vi "Main.vi"() -> ()   [LabVIEW 2024]
uses:
  AD2_WFG_SDK_class/WFG.ctl
  AD2_WFG_SDK_class/WFGCh.ctl
  AD2_WFG_SDK_class/AD2TriggerSources.ctl
  Hamamatsu_class/SubRegion.ctl
  REGLO Digital/Controlling_the_Pump_Reglo_D.ctl
  AD2_DO_SDK_class/DOConfigureCustomData.ctl
  AD2_DO_SDK_class/DOTrigger.ctl
  AD2_DO_SDK_class/DOCustomData.ctl
  Application_class/Application.lvclass
  Users/Lab user/AppData/Local/CETONI_SDK/lib/labview/labbCAN_Bus_API/SiUnitPrefix.ctl
  Users/Lab user/AppData/Local/CETONI_SDK/lib/labview/labbCAN_Bus_API/TimeUnits.ctl
  Users/Lab user/AppData/Local/CETONI_SDK/lib/labview/labbCAN_Pump_API/VolumeUnits.ctl
  CetoniPump_class/CetoniPump.lvclass
  Cetoni_Simulated_class/Cetoni_Simulated.lvclass
  C:/git/thermacoustics/CetoniPump_class/CetoniPump.lvclass
  Hamamatsu_class/Hamamatsu.lvclass
  Hamamatsu_simulated_class/Hamamatsu_simulated.lvclass
  C:/git/thermacoustics/Hamamatsu_class/Hamamatsu.lvclass
  ExperimentSeries2_class/ExperimentSeries2.lvclass
  Valve_class/Valve.lvclass
  Valve_Sim_class/Valve_Sim.lvclass
  C:/git/thermacoustics/Valve_class/Valve.lvclass
  <vilib>/Utility/error.llb/Error Cluster From Error Code.vi
  <vilib>/ErrorRing/Error Ring.xnode
  AD2_SDK_class/AD2_SDK.lvclass
  Prior_Zmotor_class/Prior_Zmotor.lvclass
  Users/Lab user/AppData/Local/CETONI_SDK/lib/labview/labbCAN_Pump_API/labbCAN_Pump_API.lvlib
  Users/Lab user/AppData/Local/CETONI_SDK/lib/labview/labbCAN_Bus_API/labbCAN_Bus_API.lvlib
  AD2_WFG_SDK_class/AD2_WFG_SDK.lvclass
  AD2_DO_SDK_class/AD2_DO_SDK.lvclass
panel:
  in  "Abort":bool
  out "Error Out":errorcluster
  in  "Tab Control":T1(tab)=enum."Experiment"
  in  "Cetoni Device Configuration Path":string="C:\\Users\\Lab user\\Desktop\\Franzi\\Cetoni_1pump_config_FM"
  in  "Valve  VISA resource name":refnum<visa-resource-name>="COM5"
  in  "Prior Visa resource name":refnum<visa-resource-name>="COM7"
  in  "Simulate Camera":bool
  in  "Simulate Valve":bool
  in  "Simulate Pump":bool
  in  "Initialize System":bool
  in  "Z stage":bool
  in  "Analog Discovery 3":bool=TRUE
  in  "Hamamatsu":bool=TRUE
  in  "Cetoni Pump":bool=TRUE
  in  "MX Valve 2":bool=TRUE
  in  "WFGConfig":T2={"Running"=TRUE, "Ch1"={"idxChannel"=0, "Settings out of range"=FALSE, "Carrier"={"Frequency (Hz)"=1975000.0, "Amplitude (V)"=2.0, "Offset(V)"=0.0, "Symmetry(%) "=50.0, "Phase(Deg)"=0.0, "Function"=1, "Enable"=FALSE}, "Trigger"={"secRun(0=Cont)"=0.0, "secWait"=0.0, "cRepeat(0=inf)"=0, "Repeat Trigger"=FALSE, "TrigrSrc"=enum."trigrsrcNone"}, "FM Mod"={"Frequency (Hz)"=1000.0, "Amplitude (%)"=1.0, "Offset(V)"=0.0, "Symmetry(%) "=50.0, "Phase(Deg)"=0.0, "Function 2"=1, "Enable"=FALSE}}, "Ch2"={"idxChannel"=1, "Settings out of range"=FALSE, "Carrier"={"Frequency (Hz)"=1000.0, "Amplitude (V)"=1.0, "Offset(V)"=0.0, "Symmetry(%) "=50.0, "Phase(Deg)"=0.0, "Function"=1, "Enable"=FALSE}, "Trigger"={"secRun(0=Cont)"=0.0, "secWait"=0.0, "cRepeat(0=inf)"=0, "Repeat Trigger"=FALSE, "TrigrSrc"=enum."trigrsrcNone"}, "FM Mod"={"Frequency (Hz)"=1000.0, "Amplitude (%)"=1.0, "Offset(V)"=0.0, "Symmetry(%) "=50.0, "Phase(Deg)"=0.0, "Function 2"=1, "Enable"=FALSE}}, "SyncronizeState"=enum."Independent"} {"Ch2"."FM Mod"."Function 2" items=["DC"=0, "Sine"=1, "Square"=2, "Triangle"=3, "RampUp"=4, "RampDown"=5, "Noise"=6, "Pulse"=7, "Custom"=30]; "Ch2"."Carrier"."Function" items=["DC"=0, "Sine"=1, "Square"=2, "Triangle"=3, "RampUp"=4, "RampDown"=5, "Noise"=6, "Pulse"=7, "Custom"=30]; "Ch1"."FM Mod"."Function 2" items=["DC"=0, "Sine"=1, "Square"=2, "Triangle"=3, "RampUp"=4, "RampDown"=5, "Noise"=6, "Pulse"=7, "Custom"=30]; "Ch1"."Carrier"."Function" items=["DC"=0, "Sine"=1, "Square"=2, "Triangle"=3, "RampUp"=4, "RampDown"=5, "Noise"=6, "Pulse"=7, "Custom"=30]; "Ch1"."Carrier"."Frequency (Hz)" step=5000.0}
  in  "Freq Sweep (Ch1)":T5
  in  "Read Pump Status":bool
  in  "Number of flushes":dbl=2.0
  in  "Valve Pos1":bool
  in  "ValvePos2":bool
  in  "Command":T6=enum."Stop Reglo Digital"
  in  "Send Pump Command":bool
  in  "Flush":bool
  in  "Refill":bool
  in  "Flow Rate":dbl=-5000.0
  in  "Go to Level":bool
  in  "Level(ml)":dbl
  in  "Generate Flow":bool
  in  "Empty":bool
  in  "ConfigureSyringe":bool
  in  "Flush":bool
  in  "Reference move":bool
  in  "Stop Syringe":bool
  in  "Syringe":T7(ring)=enum."BD 5ml"
  in  "Flush Settings":T8={"Flush Flowrate"=1000.0, "flush volume (ml)"=0.01, "WaitAfterFlush"=5.0}
  out "Fill Level":dbl
  out "Is pumping":bool
  out "Actual Flow Rate":dbl
  in  "Adjust Intensity in image":bool
  in  "Image Continous":bool=TRUE
  in  "Center ROI":bool
  in  "ExposureTime(ms)":dbl=40.0
  in  "ROI":T9={"Horizontal Offset"=0, "Vertical Offset"=792, "Horizontal Size"=2304, "Vertical Size"=740} {"Vertical Size" min=4 max=1512 step=4; "Horizontal Size" min=4 max=2304 step=4; "Vertical Offset" min=0 max=1564 step=4; "Horizontal Offset" min=0 max=0 step=4}
  in  "Image":bool
  in  "Configure Camera":bool
  in  "Trigg":bool
  out "Frame Index 2":i32
  out "Frame Count 2":i32
  in  "StartSequence":bool
  in  "SaveSequence":bool
  in  "Sequence path":path
  in  "Sequence Settings":T10={"Master Pulse Settings"={"Mode"=1, "Source"=1, "Interval"=1.0, "Burst"=0}, "Capture mode"=0, "Frames"=0, "Dcam Trigger Source"=1, "External Options"={"Polarity"=1, "Delay"=0.0}, "ExposureTime(ms)"=0.0} {"External Options"."Polarity" items=["Negative"=1, "Positive"=2]; "Dcam Trigger Source" items=["Internal"=1, "External"=2, "Software"=3, "Master Pulse"=4]; "Capture mode" items=["Snap", "Sequence"]; "Master Pulse Settings"."Source" items=["External"=1, "Software"=2]; "Master Pulse Settings"."Mode" items=["Continuous"=1, "Start"=2, "Burst"=3]}
  in  "Conversion Policy (Default)":T11={"Conversion Method"=15, "Minimum Value"=0, "Maximum Value"=0, "# Shifts"=0} {"Conversion Method" items=["Default"=10, "Most Significant Bits"=11, "Full Dynamic"=12, "Downshift"=13, "Given Range"=14, "90% Dynamic"=15, "Given Percent Range"=16]}
  in  "?":T12={"DO Trigger"={"secRun(0=Cont)"=0.0, "secWait"=0.0, "cRepeat(0=inf)"=0, "Repeat Trigger"=FALSE, "TrigrSrc"=enum."trigrsrcNone"}, "CustomData"=[{"Data"=[FALSE, TRUE, FALSE, FALSE, FALSE, FALSE, FALSE, FALSE, FALSE, FALSE, FALSE, FALSE, FALSE, FALSE, FALSE, FALSE, FALSE, FALSE, FALSE, FALSE, FALSE, FALSE], "Freq"=1000.0, "#Bits"=100, "Enable"=FALSE, "IdleState"=0}, {"Data"=[TRUE, TRUE, TRUE, TRUE, TRUE, FALSE, FALSE, FALSE, FALSE, FALSE, FALSE, FALSE, FALSE, FALSE, FALSE, FALSE, FALSE, FALSE, FALSE, FALSE, FALSE, FALSE], "Freq"=1000.0, "#Bits"=100, "Enable"=FALSE, "IdleState"=0}, {"Data"=[], "Freq"=0.0, "#Bits"=0, "Enable"=FALSE, "IdleState"=0}, {"Data"=[FALSE, FALSE, FALSE, FALSE, FALSE, FALSE, FALSE, FALSE, FALSE, FALSE, FALSE, FALSE, FALSE, FALSE, FALSE, FALSE, FALSE, FALSE, FALSE, FALSE, FALSE, FALSE, FALSE], "Freq"=0.0, "#Bits"=0, "Enable"=FALSE, "IdleState"=0}, {"Data"=[], "Freq"=0.0, "#Bits"=0, "Enable"=FALSE, "IdleState"=0}, {"Data"=[], "Freq"=0.0, "#Bits"=0, "Enable"=FALSE, "IdleState"=0}, {"Data"=[], "Freq"=0.0, "#Bits"=0, "Enable"=FALSE, "IdleState"=0}, {"Data"=[], "Freq"=0.0, "#Bits"=0, "Enable"=FALSE, "IdleState"=0}, {"Data"=[], "Freq"=0.0, "#Bits"=0, "Enable"=FALSE, "IdleState"=0}, {"Data"=[], "Freq"=0.0, "#Bits"=0, "Enable"=FALSE, "IdleState"=0}, {"Data"=[], "Freq"=0.0, "#Bits"=0, "Enable"=FALSE, "IdleState"=0}, {"Data"=[], "Freq"=0.0, "#Bits"=0, "Enable"=FALSE, "IdleState"=0}, {"Data"=[], "Freq"=0.0, "#Bits"=0, "Enable"=FALSE, "IdleState"=0}, {"Data"=[], "Freq"=0.0, "#Bits"=0, "Enable"=FALSE, "IdleState"=0}, {"Data"=[], "Freq"=0.0, "#Bits"=0, "Enable"=FALSE, "IdleState"=0}, {"Data"=[FALSE, FALSE, FALSE, FALSE, FALSE, FALSE, FALSE, FALSE, FALSE, FALSE, FALSE, FALSE, FALSE, FALSE, FALSE, FALSE, FALSE, FALSE, FALSE, FALSE, FALSE, FALSE, FALSE], "Freq"=0.0, "#Bits"=0, "Enable"=FALSE, "IdleState"=0}, {"Data"=[FALSE, FALSE, FALSE, FALSE, FALSE, FALSE, FALSE, FALSE, FALSE, FALSE, FALSE, FALSE, FALSE, FALSE, FALSE, FALSE, FALSE, FALSE, FALSE, FALSE, FALSE, FALSE, FALSE], "Freq"=0.0, "#Bits"=0, "Enable"=FALSE, "IdleState"=0}]}
  in  "Configure DO":bool
  in  "Configure DO Clock":bool
  in  "DO Trigger":T13
  in  "ClockSettings":T15(array[cluster])
  in  "TriggAD2":bool
  in  "Frequency List Generator":bool
  in  "Frequency List":dbl[](array[numeric])=[0.0, 1.0]
  in  "Dynamic Frequency \n(or center freq)":bool
  in  "SeriesPath 2":path=path "D:/2026-02-17_Rev_Strea_OffcLaser_1micr/1975kHz/1500mMol_20C_test2"
  in  "Start Experiment series":bool
  out "# elements in queue":i32=1
  out "Time Left":dbl=inf format="%<%H:%M:%S>t"
  out "Elapsed Time":dbl=6.602530002593994 format="%<%H:%M:%S>t"
  in  "Frames":i32=1000 min=1
  in  "ExposureTime(ms) 2":dbl=40.0
  in  "Repeats":i32=1 min=1
  in  "Flush Settings 2":T16={"Flush Flowrate(uL)"=1000.0, "flush volume (ml)"=0.01, "WaitAfterFlush"=2.0}
  out "Waveform Graph":dbl[](graph)=[0.04999995231628418, 0.05000019073486328, 0.050000905990600586, 0.04999995231628418, 0.05000114440917969, 0.04999995231628418, 0.050000905990600586, 0.04999995231628418, 0.05000114440917969, 0.04999995231628418, 0.050000905990600586, 0.05000019073486328, 0.050000905990600586, 0.04999995231628418, 0.05000114440917969, 0.04999995231628418, 0.050000905990600586, 0.04999995231628418, 0.049996137619018555, 0.04999995231628418, 0.050000905990600586, 0.05000019073486328, 0.04999995231628418, 0.050000905990600586, 0.04999995231628418, 0.05000114440917969, 0.04999995231628418, 0.050000905990600586, 0.05000019073486328, 0.050000905990600586, 0.04999995231628418, 0.05000114440917969, 0.04999995231628418, 0.050000905990600586, 0.04999995231628418, 0.05000114440917969, 0.04999995231628418, 0.050000905990600586, 0.05000019073486328, 0.04999589920043945, 0.04999995231628418, 0.05000114440917969, 0.04999995231628418, 0.04999995231628418, 0.050000905990600586, 0.05000019073486328, 0.050000905990600586, 0.04999995231628418, 0.05000114440917969, 0.04999995231628418, 0.050000905990600586, 0.04999995231628418, 0.05000114440917969, 0.04999995231628418, 0.050000905990600586, 0.05000019073486328, 0.050000905990600586, 0.04999995231628418, 0.05000114440917969, 0.04999995231628418, 0.04999589920043945, 0.04999995231628418, 0.05000114440917969, 0.04999995231628418, 0.04999995231628418, 0.05000114440917969, 0.04999995231628418, 0.050000905990600586, 0.04999995231628418, 0.05000114440917969, 0.04999995231628418, 0.050000905990600586, 0.05000019073486328, 0.050000905990600586, 0.04999995231628418, 0.050000905990600586, 0.05000019073486328, 0.050000905990600586, 0.04999995231628418, 0.05000114440917969, 0.04999995231628418, 0.04999589920043945, 0.05000019073486328, 0.050000905990600586, 0.04999995231628418, 0.050000905990600586, 0.05000019073486328, 0.04999995231628418, 0.050000905990600586, 0.04999995231628418, 0.05000114440917969, 0.04999995231628418, 0.050000905990600586, 0.05000019073486328, 0.050000905990600586, 0.04999995231628418, 0.05000114440917969, 0.04999995231628418, 0.050000905990600586, 0.04999995231628418, 0.05000114440917969, 0.04999995231628418, 0.04999589920043945, 0.05000019073486328, 0.050000905990600586, 0.04999995231628418, 0.05000114440917969, 0.04999995231628418, 0.04999995231628418, 0.050000905990600586, 0.05000019073486328, 0.050000905990600586, 0.04999995231628418, 0.05000114440917969, 0.04999995231628418, 0.050000905990600586, 0.04999995231628418, 0.05000114440917969, 0.04999995231628418, 0.050000905990600586, 0.05000019073486328, 0.050000905990600586, 0.04999995231628418, 0.049996137619018555, 0.04999995231628418, 0.050000905990600586, 0.04999995231628418, 0.05000114440917969, 0.04999995231628418, 0.04999995231628418, 0.05000114440917969, 0.04999995231628418, 0.050000905990600586, 0.04999995231628418, 0.05000114440917969, 0.04999995231628418, 0.050000905990600586, 0.05000019073486328, 0.050000905990600586, 0.04999995231628418, 0.05000114440917969, 0.04999995231628418, 0.050000905990600586, 0.04999494552612305, 0.05000114440917969, 0.04999995231628418, 0.050000905990600586, 0.05000019073486328, 0.050000905990600586, 0.04999995231628418, 0.04999995231628418, 0.05000114440917969, 0.04999995231628418, 0.050000905990600586, 0.05000019073486328, 0.050000905990600586, 0.04999995231628418, 0.05000114440917969, 0.04999995231628418, 0.050000905990600586, 0.04999995231628418, 0.05000114440917969, 0.04999995231628418, 0.050000905990600586, 0.04999518394470215, 0.050000905990600586, 0.04999995231628418, 0.05000114440917969, 0.04999995231628418, 0.050000905990600586, 0.04999995231628418, 0.05000114440917969, 0.04999995231628418, 0.04999995231628418, 0.05000114440917969, 0.04999995231628418, 0.050000905990600586, 0.04999995231628418, 0.05000114440917969, 0.04999995231628418, 0.050000905990600586, 0.05000019073486328, 0.050000905990600586, 0.04999995231628418, 0.05000114440917969, 0.04999494552612305, 0.050000905990600586, 0.04999995231628418, 0.05000114440917969, 0.04999995231628418, 0.050000905990600586, 0.05000019073486328, 0.050000905990600586, 0.04999995231628418, 0.04999995231628418, 0.05000114440917969, 0.04999995231628418, 0.050000905990600586, 0.05000019073486328, 0.050000905990600586, 0.04999995231628418, 0.05000114440917969, 0.04999995231628418, 0.050000905990600586, 0.04999995231628418, 0.049996137619018555, 0.04999995231628418, 0.050000905990600586, 0.05000019073486328, 0.050000905990600586, 0.04999995231628418, 0.05000114440917969, 0.04999995231628418, 0.050000905990600586, 0.04999995231628418, 0.05000019073486328, 0.050000905990600586, 0.04999995231628418, 0.05000114440917969, 0.04999995231628418, 0.050000905990600586, 0.04999995231628418, 0.05000114440917969, 0.04999995231628418, 0.050000905990600586, 0.04999518394470215, 0.050000905990600586, 0.04999995231628418, 0.05000114440917969, 0.04999995231628418, 0.050000905990600586, 0.04999995231628418, 0.05000114440917969, 0.04999995231628418, 0.050000905990600586, 0.04999995231628418, 0.05000019073486328, 0.050000905990600586, 0.04999995231628418, 0.05000114440917969, 0.04999995231628418, 0.050000905990600586, 0.04999995231628418, 0.05000114440917969, 0.04999995231628418, 0.04999589920043945, 0.05000019073486328, 0.050000905990600586, 0.04999995231628418, 0.05000114440917969, 0.04999995231628418, 0.050000905990600586, 0.04999995231628418, 0.05000114440917969, 0.04999995231628418, 0.050000905990600586, 0.05000019073486328, 0.050000905990600586, 0.04999995231628418, 0.04999995231628418, 0.05000114440917969, 0.04999995231628418, 0.050000905990600586, 0.05000019073486328, 0.050000905990600586, 0.04999995231628418, 0.049996137619018555, 0.04999995231628418, 0.050000905990600586, 0.04999995231628418, 0.05000114440917969, 0.04999995231628418, 0.050000905990600586, 0.05000019073486328, 0.050000905990600586, 0.04999995231628418, 0.05000114440917969, 0.04999995231628418, 0.050000905990600586, 0.04999995231628418, 0.05000019073486328, 0.050000905990600586, 0.04999995231628418, 0.05000114440917969, 0.04999995231628418, 0.050000905990600586, 0.04999995231628418, 0.049996137619018555, 0.04999995231628418, 0.050000905990600586, 0.05000019073486328, 0.050000905990600586, 0.04999995231628418, 0.05000114440917969, 0.04999995231628418, 0.050000905990600586, 0.04999995231628418, 0.05000114440917969, 0.04999995231628418, 0.050000905990600586, 0.05000019073486328, 0.04999995231628418, 0.050000905990600586, 0.04999995231628418, 0.05000114440917969, 0.04999995231628418, 0.050000905990600586, 0.05000019073486328, 0.04999589920043945, 0.04999995231628418, 0.05000114440917969, 0.04999995231628418, 0.050000905990600586, 0.04999995231628418, 0.05000114440917969, 0.04999995231628418, 0.050000905990600586, 0.05000019073486328, 0.050000905990600586, 0.04999995231628418, 0.05000114440917969, 0.04999995231628418, 0.04999995231628418, 0.050000905990600586, 0.05000019073486328, 0.050000905990600586, 0.04999995231628418, 0.05000114440917969, 0.04999494552612305, 0.050000905990600586, 0.04999995231628418, 0.05000114440917969, 0.04999995231628418, 0.050000905990600586, 0.05000019073486328, 0.050000905990600586, 0.04999995231628418, 0.05000114440917969, 0.04999995231628418, 0.050000905990600586, 0.04999995231628418, 0.05000114440917969, 0.04999995231628418, 0.050000905990600586, 0.05000019073486328, 0.04999995231628418, 0.050000905990600586, 0.04999995231628418, 0.05000114440917969, 0.04999494552612305, 0.050000905990600586, 0.05000019073486328, 0.050000905990600586, 0.04999995231628418, 0.05000114440917969, 0.04999995231628418, 0.050000905990600586, 0.04999995231628418, 0.05000114440917969, 0.04999995231628418, 0.050000905990600586, 0.05000019073486328, 0.050000905990600586, 0.04999995231628418, 0.05000114440917969, 0.04999995231628418, 0.04999995231628418, 0.050000905990600586, 0.04999995231628418, 0.049996137619018555, 0.04999995231628418, 0.05000114440917969, 0.04999995231628418, 0.050000905990600586, 0.04999995231628418, 0.05000114440917969, 0.04999995231628418, 0.050000905990600586, 0.04999995231628418, 0.05000114440917969, 0.04999995231628418, 0.050000905990600586, 0.05000019073486328, 0.050000905990600586, 0.04999995231628418, 0.05000114440917969, 0.04999995231628418, 0.04999995231628418, 0.050000905990600586, 0.05000019073486328, 0.04999589920043945, 0.04999995231628418, 0.05000114440917969, 0.04999995231628418, 0.050000905990600586, 0.04999995231628418, 0.05000114440917969, 0.04999995231628418, 0.050000905990600586, 0.05000019073486328, 0.050000905990600586, 0.04999995231628418, 0.05000114440917969, 0.04999995231628418, 0.050000905990600586, 0.04999995231628418, 0.05000114440917969, 0.04999995231628418, 0.04999995231628418, 0.05000114440917969, 0.04999995231628418, 0.050000905990600586, 0.049996137619018555, 0.04999995231628418, 0.04999995231628418, 0.050000905990600586, 0.05000019073486328, 0.050000905990600586, 0.04999995231628418, 0.05000114440917969, 0.04999995231628418, 0.050000905990600586, 0.04999995231628418, 0.05000114440917969, 0.04999995231628418, 0.050000905990600586, 0.05000019073486328, 0.050000905990600586, 0.04999995231628418, 0.05000114440917969, 0.04999995231628418, 0.04999995231628418, 0.050000905990600586, 0.049996137619018555, 0.04999995231628418, 0.04999995231628418, 0.05000114440917969, 0.04999995231628418, 0.050000905990600586, 0.04999995231628418, 0.05000114440917969, 0.04999995231628418, 0.050000905990600586, 0.05000019073486328, 0.050000905990600586, 0.04999995231628418, 0.05000114440917969, 0.04999995231628418, 0.050000905990600586, 0.04999995231628418, 0.05000114440917969, 0.04999995231628418, 0.04999995231628418, 0.05000114440917969, 0.04999589920043945, 0.04999995231628418, 0.04999995231628418, 0.05000114440917969, 0.04999995231628418, 0.050000905990600586, 0.05000019073486328, 0.050000905990600586, 0.04999995231628418, 0.05000114440917969, 0.04999995231628418, 0.050000905990600586, 0.04999995231628418, 0.05000114440917969, 0.04999995231628418, 0.050000905990600586, 0.05000019073486328, 0.050000905990600586, 0.04999995231628418, 0.04999995231628418, 0.049996137619018555, 0.050000905990600586, 0.04999995231628418, 0.05000019073486328, 0.050000905990600586, 0.04999995231628418, 0.05000114440917969, 0.04999995231628418, 0.050000905990600586, 0.04999995231628418, 0.05000114440917969, 0.04999995231628418, 0.050000905990600586, 0.05000019073486328, 0.050000905990600586, 0.04999995231628418, 0.05000114440917969, 0.04999995231628418, 0.050000905990600586, 0.04999995231628418, 0.05000019073486328, 0.04999589920043945, 0.050000905990600586, 0.05000019073486328, 0.050000905990600586, 0.04999995231628418, 0.04999995231628418, 0.05000114440917969, 0.04999995231628418, 0.050000905990600586, 0.05000019073486328, 0.050000905990600586, 0.04999995231628418, 0.05000114440917969, 0.04999995231628418, 0.050000905990600586, 0.04999995231628418, 0.05000114440917969, 0.04999995231628418, 0.050000905990600586, 0.04999995231628418, 0.05000114440917969, 0.04999494552612305, 0.05000114440917969, 0.04999995231628418, 0.050000905990600586, 0.04999995231628418, 0.05000019073486328, 0.050000905990600586, 0.04999995231628418, 0.050000905990600586, 0.05000019073486328, 0.050000905990600586, 0.04999995231628418, 0.05000114440917969, 0.04999995231628418, 0.050000905990600586, 0.04999995231628418, 0.05000114440917969, 0.04999995231628418, 0.050000905990600586, 0.05000019073486328, 0.050000905990600586, 0.04999494552612305, 0.05000114440917969, 0.04999995231628418, 0.050000905990600586, 0.04999995231628418, 0.05000019073486328, 0.050000905990600586, 0.04999995231628418, 0.05000114440917969, 0.04999995231628418, 0.050000905990600586, 0.04999995231628418, 0.05000114440917969, 0.04999995231628418, 0.050000905990600586, 0.05000019073486328, 0.050000905990600586, 0.04999995231628418, 0.05000114440917969, 0.04999995231628418, 0.050000905990600586, 0.04999995231628418, 0.049996137619018555, 0.04999995231628418, 0.050000905990600586, 0.05000019073486328, 0.04999995231628418, 0.050000905990600586, 0.04999995231628418, 0.05000114440917969, 0.04999995231628418, 0.050000905990600586, 0.05000019073486328, 0.050000905990600586, 0.04999995231628418, 0.05000114440917969, 0.04999995231628418, 0.050000905990600586, 0.04999995231628418, 0.05000114440917969, 0.04999995231628418, 0.050000905990600586, 0.05000019073486328, 0.04999589920043945, 0.04999995231628418, 0.05000114440917969, 0.04999995231628418, 0.050000905990600586, 0.04999995231628418, 0.05000019073486328, 0.050000905990600586, 0.04999995231628418, 0.05000114440917969, 0.04999995231628418, 0.050000905990600586, 0.04999995231628418, 0.05000114440917969, 0.04999995231628418, 0.050000905990600586, 0.05000019073486328, 0.050000905990600586, 0.04999995231628418, 0.05000114440917969, 0.04999995231628418, 0.050000905990600586, 0.04999494552612305, 0.05000114440917969, 0.04999995231628418, 0.050000905990600586, 0.05000019073486328, 0.04999995231628418, 0.050000905990600586, 0.04999995231628418, 0.05000114440917969, 0.04999995231628418, 0.050000905990600586, 0.05000019073486328, 0.050000905990600586, 0.04999995231628418, 0.05000114440917969, 0.04999995231628418, 0.050000905990600586, 0.04999995231628418, 0.05000114440917969, 0.04999995231628418, 0.050000905990600586, 0.05000019073486328, 0.04999589920043945, 0.04999995231628418, 0.05000114440917969, 0.04999995231628418, 0.04999995231628418, 0.050000905990600586, 0.05000019073486328, 0.050000905990600586, 0.04999995231628418, 0.05000114440917969, 0.04999995231628418, 0.050000905990600586, 0.04999995231628418, 0.05000114440917969, 0.04999995231628418, 0.050000905990600586, 0.05000019073486328, 0.050000905990600586, 0.04999995231628418, 0.05000114440917969, 0.04999995231628418, 0.04999589920043945, 0.04999995231628418, 0.05000114440917969, 0.04999995231628418, 0.04999995231628418, 0.05000114440917969, 0.04999995231628418, 0.050000905990600586, 0.04999995231628418, 0.05000114440917969, 0.04999995231628418, 0.050000905990600586, 0.05000019073486328, 0.050000905990600586, 0.04999995231628418, 0.050000905990600586, 0.05000019073486328, 0.050000905990600586, 0.04999995231628418, 0.05000114440917969, 0.04999995231628418, 0.04999589920043945, 0.05000019073486328, 0.050000905990600586, 0.04999995231628418, 0.050000905990600586, 0.05000019073486328, 0.04999995231628418, 0.050000905990600586, 0.04999995231628418, 0.05000114440917969, 0.04999995231628418, 0.050000905990600586, 0.05000019073486328, 0.050000905990600586, 0.04999995231628418, 0.05000114440917969, 0.04999995231628418, 0.050000905990600586, 0.04999995231628418, 0.05000114440917969, 0.04999995231628418, 0.04999589920043945, 0.05000019073486328, 0.050000905990600586, 0.04999995231628418, 0.05000114440917969, 0.04999995231628418, 0.04999995231628418, 0.050000905990600586, 0.05000019073486328, 0.050000905990600586, 0.04999995231628418, 0.05000114440917969, 0.04999995231628418, 0.050000905990600586, 0.04999995231628418, 0.05000114440917969, 0.04999995231628418, 0.050000905990600586, 0.05000019073486328, 0.050000905990600586, 0.04999995231628418, 0.049996137619018555, 0.04999995231628418, 0.050000905990600586, 0.04999995231628418, 0.05000114440917969, 0.04999995231628418, 0.04999995231628418, 0.05000114440917969, 0.04999995231628418, 0.050000905990600586, 0.04999995231628418, 0.05000114440917969, 0.04999995231628418, 0.050000905990600586, 0.05000019073486328, 0.050000905990600586, 0.04999995231628418, 0.05000114440917969, 0.04999995231628418, 0.050000905990600586, 0.04999995231628418, 0.049996137619018555, 0.04999995231628418, 0.050000905990600586, 0.05000019073486328, 0.050000905990600586, 0.04999995231628418, 0.04999995231628418, 0.05000114440917969, 0.04999995231628418, 0.050000905990600586, 0.05000019073486328, 0.050000905990600586, 0.04999995231628418, 0.05000114440917969, 0.04999995231628418, 0.050000905990600586, 0.04999995231628418, 0.05000114440917969, 0.04999995231628418, 0.050000905990600586, 0.04999518394470215, 0.050000905990600586, 0.04999995231628418, 0.05000114440917969, 0.04999995231628418, 0.050000905990600586, 0.04999995231628418, 0.05000114440917969, 0.04999995231628418, 0.04999995231628418, 0.05000114440917969, 0.04999995231628418, 0.050000905990600586, 0.04999995231628418, 0.05000114440917969, 0.04999995231628418, 0.050000905990600586, 0.05000019073486328, 0.050000905990600586, 0.04999995231628418, 0.05000114440917969, 0.04999494552612305, 0.050000905990600586, 0.04999995231628418, 0.05000114440917969, 0.04999995231628418, 0.050000905990600586, 0.05000019073486328, 0.050000905990600586, 0.04999995231628418, 0.04999995231628418, 0.05000114440917969, 0.04999995231628418, 0.050000905990600586, 0.05000019073486328, 0.050000905990600586, 0.04999995231628418, 0.05000114440917969, 0.04999995231628418, 0.050000905990600586, 0.04999995231628418, 0.049996137619018555, 0.04999995231628418, 0.050000905990600586, 0.05000019073486328, 0.050000905990600586, 0.04999995231628418, 0.05000114440917969, 0.04999995231628418, 0.050000905990600586, 0.04999995231628418, 0.05000019073486328, 0.050000905990600586, 0.04999995231628418, 0.05000114440917969, 0.04999995231628418, 0.050000905990600586, 0.04999995231628418, 0.05000114440917969, 0.04999995231628418, 0.050000905990600586, 0.04999995231628418, 0.049996137619018555, 0.04999995231628418, 0.05000114440917969, 0.04999995231628418, 0.050000905990600586, 0.04999995231628418, 0.05000114440917969, 0.04999995231628418, 0.050000905990600586, 0.04999995231628418, 0.05000019073486328, 0.050000905990600586, 0.04999995231628418, 0.05000114440917969, 0.04999995231628418, 0.050000905990600586, 0.04999995231628418, 0.05000114440917969, 0.04999995231628418, 0.050000905990600586, 0.05000019073486328, 0.04999589920043945, 0.04999995231628418, 0.05000114440917969, 0.04999995231628418, 0.050000905990600586, 0.04999995231628418, 0.05000114440917969, 0.04999995231628418, 0.050000905990600586, 0.05000019073486328, 0.050000905990600586, 0.04999995231628418, 0.04999995231628418, 0.05000114440917969, 0.04999995231628418, 0.050000905990600586, 0.05000019073486328, 0.050000905990600586, 0.04999995231628418, 0.05000114440917969, 0.04999995231628418, 0.04999589920043945, 0.04999995231628418, 0.05000114440917969, 0.04999995231628418, 0.050000905990600586, 0.05000019073486328, 0.050000905990600586, 0.04999995231628418, 0.05000114440917969, 0.04999995231628418, 0.050000905990600586, 0.04999995231628418, 0.05000019073486328, 0.050000905990600586, 0.04999995231628418, 0.05000114440917969, 0.04999995231628418, 0.050000905990600586, 0.04999995231628418, 0.049996137619018555, 0.04999995231628418, 0.050000905990600586, 0.05000019073486328, 0.050000905990600586, 0.04999995231628418, 0.05000114440917969, 0.04999995231628418, 0.050000905990600586, 0.04999995231628418, 0.05000114440917969, 0.04999995231628418, 0.050000905990600586, 0.05000019073486328, 0.04999995231628418, 0.050000905990600586, 0.04999995231628418, 0.05000114440917969, 0.04999995231628418, 0.050000905990600586, 0.04999518394470215, 0.050000905990600586, 0.04999995231628418, 0.05000114440917969, 0.04999995231628418, 0.050000905990600586, 0.04999995231628418, 0.05000114440917969, 0.04999995231628418, 0.050000905990600586, 0.05000019073486328, 0.050000905990600586, 0.04999995231628418, 0.05000114440917969, 0.04999995231628418, 0.04999995231628418, 0.050000905990600586, 0.05000019073486328, 0.050000905990600586, 0.04999995231628418, 0.049996137619018555, 0.04999995231628418, 0.050000905990600586, 0.04999995231628418, 0.05000114440917969, 0.04999995231628418, 0.050000905990600586, 0.05000019073486328, 0.050000905990600586, 0.04999995231628418, 0.05000114440917969, 0.04999995231628418, 0.050000905990600586, 0.04999995231628418, 0.05000114440917969, 0.04999995231628418, 0.050000905990600586, 0.05000019073486328, 0.04999995231628418, 0.04999589920043945, 0.05000114440917969, 0.04999995231628418, 0.04999995231628418, 0.050000905990600586, 0.05000019073486328, 0.050000905990600586, 0.04999995231628418, 0.05000114440917969, 0.04999995231628418, 0.050000905990600586, 0.04999995231628418, 0.05000114440917969, 0.04999995231628418, 0.050000905990600586, 0.05000019073486328, 0.050000905990600586, 0.04999995231628418, 0.05000114440917969, 0.04999995231628418, 0.04999995231628418, 0.04999589920043945, 0.05000114440917969, 0.04999995231628418, 0.04999995231628418, 0.05000114440917969, 0.04999995231628418, 0.050000905990600586, 0.04999995231628418, 0.05000114440917969, 0.04999995231628418, 0.050000905990600586, 0.05000019073486328, 0.050000905990600586, 0.04999995231628418, 0.050000905990600586, 0.05000019073486328, 0.050000905990600586, 0.04999995231628418, 0.05000114440917969, 0.04999995231628418, 0.04999589920043945, 0.05000019073486328, 0.050000905990600586, 0.04999995231628418, 0.04999995231628418, 0.05000114440917969, 0.04999995231628418, 0.050000905990600586, 0.04999995231628418, 0.05000114440917969, 0.04999995231628418, 0.050000905990600586, 0.05000019073486328, 0.050000905990600586, 0.04999995231628418, 0.05000114440917969, 0.04999995231628418, 0.050000905990600586, 0.04999995231628418, 0.05000114440917969, 0.04999995231628418, 0.04999995231628418, 0.049996137619018555, 0.050000905990600586, 0.04999995231628418, 0.05000114440917969, 0.04999995231628418]
  out "Average FPS":dbl=20.019925398487086
  in  "Analog Discovery Settings":T17={"Camera FPS"=20.0, "Camera Start (s)"=0.0, "Ch1 Frequency (Hz)"=1975000.0, "Ch1.Carrier.Amplitude (V)"=2.0, "Ch1 Start (s)"=0.0, "Ch1 Run (s) (0=Cont)"=60.0, "Ch2 Start(s)"=0.0, "Ch2 Run (s)(0=Cont)"=60.0}
  in  "GlobalExposure":bool
  in  "Dynamic Camera Start Time":bool
  in  "Camera Start Array(s)":dbl[](array[numeric])=[0.0, 1.0]
  in  "Freq Sweep (Ch1) 2":T5
  in  "Get Z Stack":bool
  in  "GoToPosPrior":bool
  in  "Pos (um)":i32
  in  "Read Position":bool
  in  "Top":dbl
  in  "Bottom":dbl
  in  "Step Size":dbl
  in  "Zero Z":bool
  out "Position (um)":dbl
  out "Status":string="FlushComplete"
  in  "Exit":bool
  # "If Freq Sweep Is enabled, it overrides ch1 frequency"
  # "Sweep Span=Freq Stop-Freq Start\nFreq start=Center Freq- 1/2 Freq Span\nCenter Freq = Ch1 Freq or Frequency List"
  # "These Go MAX flow!"
  # "476 is Vertical is max for 100 fps"
  # "0 init\n1 low\n2 high\n3 tristate"
  # "Sweep Span=Freq Stop-Freq Start\nFreq start=Center Freq- 1/2 Freq Span\nCenter Freq = Ch1 Freq or Frequency List"
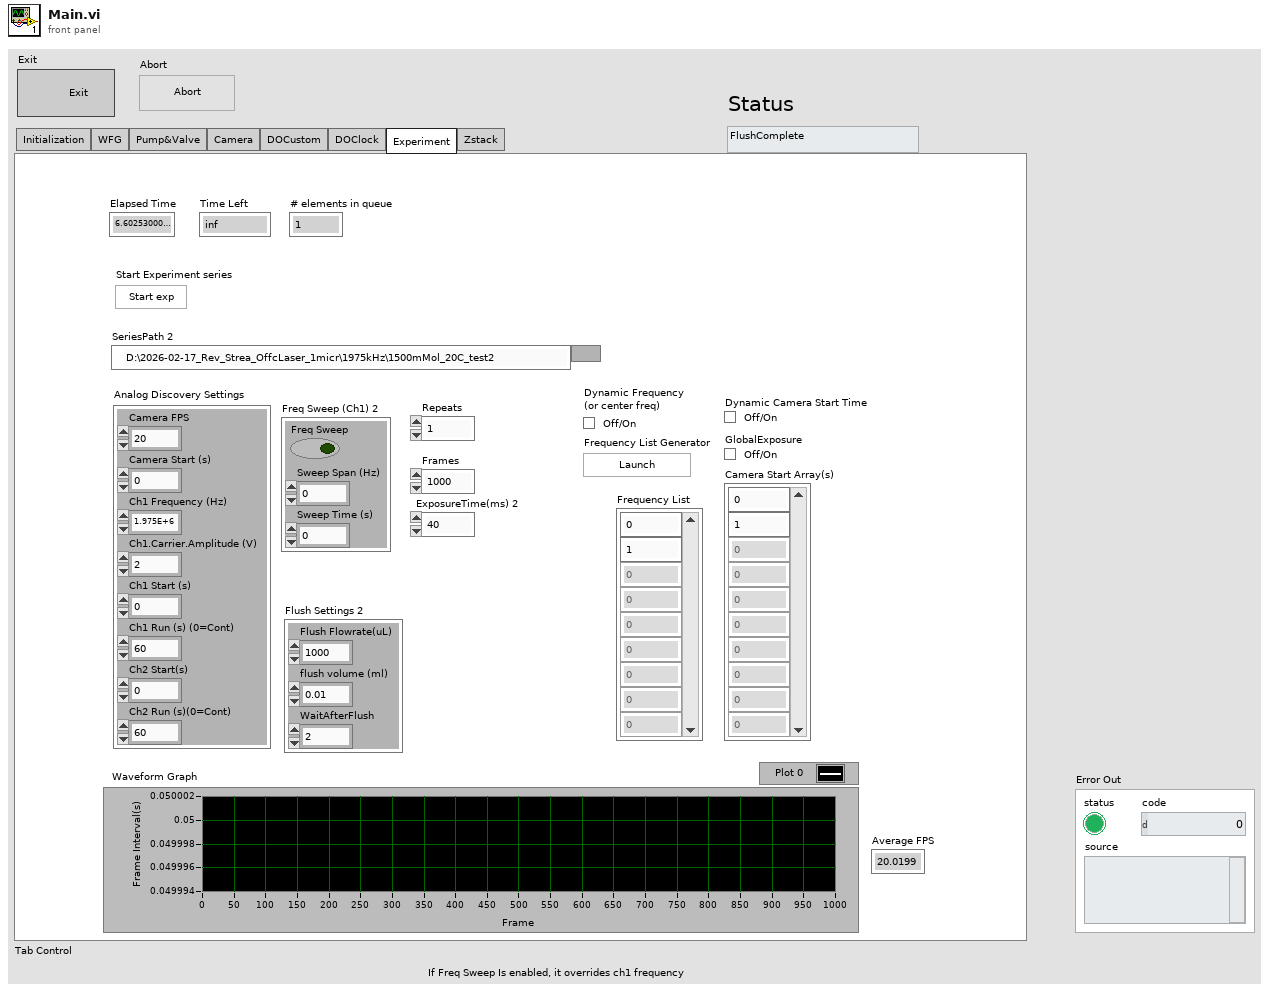
[diagram p1: front panel]
types:
  T1 = enum32{"Initialization", "WFG", "Pump&Valve", "Camera", "DOCustom", "DOClock", "Experiment", "Zstack"}
  T2 = typedef "AD2_WFG_SDK.lvclass/WFG.ctl" = cluster{"Running":bool, "Ch1":T3, "Ch2":T3, "SyncronizeState":enum16{"Independent", "Ch1Master", "Ch2Master"}}
  T3 = typedef "AD2_WFG_SDK.lvclass/WFGCh.ctl" = cluster{"idxChannel":i32, "Settings out of range":bool, "Carrier":cluster{"Frequency (Hz)":dbl, "Amplitude (V)":dbl, "Offset(V)":dbl, "Symmetry(%) ":dbl, "Phase(Deg)":dbl, "Function":u16, "Enable":bool}, "Trigger":cluster{"secRun(0=Cont)":dbl, "secWait":dbl, "cRepeat(0=inf)":i32, "Repeat Trigger":bool, "TrigrSrc":T4}, "FM Mod":cluster{"Frequency (Hz)":dbl, "Amplitude (%)":dbl, "Offset(V)":dbl, "Symmetry(%) ":dbl, "Phase(Deg)":dbl, "Function 2":u16, "Enable":bool}}
  T4 = typedef "AD2_SDK.lvclass/AD2TriggerSources.ctl" = enum8{"trigrsrcNone", "trigsrcPC", "trigsrcDetectorAnalogIn", "trigsrcDetectorDigitalIn", "trigsrcAnalogIn", "trigsrcDigitalIn", "trigsrcDigitalOut", "trigsrcAnalogOut1", "trigsrcAnalogOut2", "trigsrcAnalogOut3", "trigsrcAnalogOut4", "trigsrcExternal1", "trigsrcExternal2", "trigsrcExternal3", "trigsrcExternal4", ""}
  T5 = cluster{"Freq Sweep":bool, "Sweep Span (Hz)":dbl, "Sweep Time (s)":dbl}
  T6 = typedef "Controlling_the_Pump_Reglo_D.ctl" = enum16{"Reset overload", "Start Reglo Digital", "Stop Reglo Digital", "Revolution Clockwise", "Revolution Counter Clock Wise", "Controlpanel to Manual operation", "Controlpanel Inactiv", "Writing Numbers for Control Panel", "Writing Letters for Controlpanel"}
  T7 = enum16{"BD 1ml", "BD 3ml", "BD 5ml", "BD 10ml", "BD 20ml", "BD 30ml", "BD 50ml", "HSW 1ml"}
  T8 = cluster{"Flush Flowrate":dbl, "flush volume (ml)":dbl, "WaitAfterFlush":dbl}
  T9 = typedef "Hamamatsu.lvclass/SubRegion.ctl" = cluster{"Horizontal Offset":i32, "Vertical Offset":i32, "Horizontal Size":i32, "Vertical Size":i32}
  T10 = cluster{"Master Pulse Settings":cluster{"Mode":u32, "Source":u32, "Interval":dbl, "Burst":u32}, "Capture mode":i32, "Frames":i32, "Dcam Trigger Source":i32, "External Options":cluster{"Polarity":i32, "Delay":dbl}, "ExposureTime(ms)":dbl}
  T11 = cluster{"Conversion Method":u32, "Minimum Value":i32, "Maximum Value":i32, "# Shifts":i32}
  T12 = typedef "DOConfigureCustomData.ctl" = cluster{"DO Trigger":T13, "CustomData":T14}
  T13 = typedef "AD2_DO_SDK.lvclass/DOTrigger.ctl" = cluster{"secRun(0=Cont)":dbl, "secWait":dbl, "cRepeat(0=inf)":i32, "Repeat Trigger":bool, "TrigrSrc":T4}
  T14 = typedef "AD2_DO_SDK.lvclass/DOCustomData.ctl" = cluster{"Data":bool[], "Freq":dbl, "#Bits":u32, "Enable":bool, "IdleState":u16}[]
  T15 = cluster{"Frequency":dbl, "Enable":bool, "IdleState":enum16{"Initial", "Low", "High", "Z"}}[]
  T16 = cluster{"Flush Flowrate(uL)":dbl, "flush volume (ml)":dbl, "WaitAfterFlush":dbl}
  T17 = cluster{"Camera FPS":dbl, "Camera Start (s)":dbl, "Ch1 Frequency (Hz)":dbl, "Ch1.Carrier.Amplitude (V)":dbl, "Ch1 Start (s)":dbl, "Ch1 Run (s) (0=Cont)":dbl, "Ch2 Start(s)":dbl, "Ch2 Run (s)(0=Cont)":dbl}
  T18 = typedef "labbCAN_Bus_API.lvlib/SiUnitPrefix.ctl" = i32
  T19 = typedef "labbCAN_Bus_API.lvlib/TimeUnits.ctl" = i32
  T20 = typedef "labbCAN_Pump_API.lvlib/VolumeUnits.ctl" = i32
  T21 = cluster{"Prefix":T18, "TimeUnit":T19, "VolumeUnit":T20}
  T22 = typedef "Hamamatsu.lvclass/SubRegionLimits.ctl" = cluster{"H Offset":cluster{"Value":i32, "Limits":T23}, "V Offset":cluster{"Value":i32, "Limits":T23}, "H Size":cluster{"Value":i32, "Limits":T23}, "V Size":cluster{"Value":i32, "Limits":T23}}
  T23 = typedef "LVMinMaxIncTypeDef.ctl" = cluster{"Minimum":dbl, "Maximum":dbl, "Increment":dbl}
  T24 = cluster{"H Offset":cluster{"Value":i32, "Limits":T23}, "V Offset":cluster{"Value":i32, "Limits":T23}, "H Size":cluster{"Value":i32, "Limits":T23}, "V Size":cluster{"Value":i32, "Limits":T23}}
  T25 = typedef "IMAQ Image.ctl" = refnum<image>
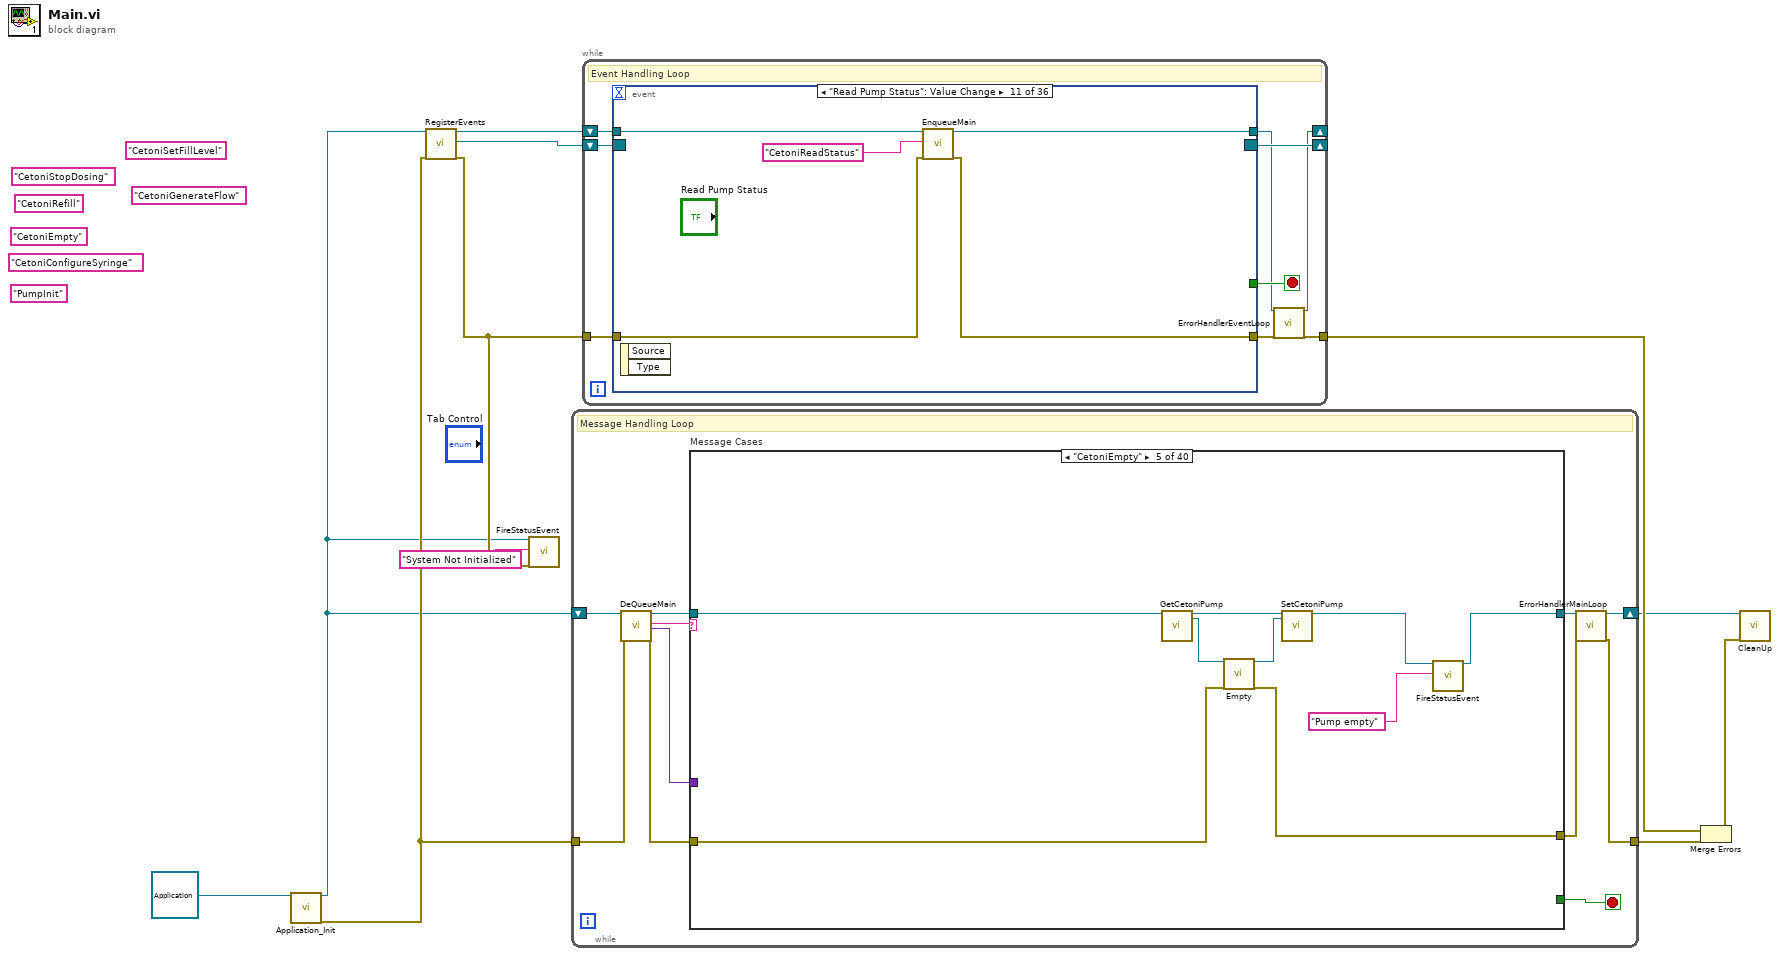
[diagram p0: block diagram]
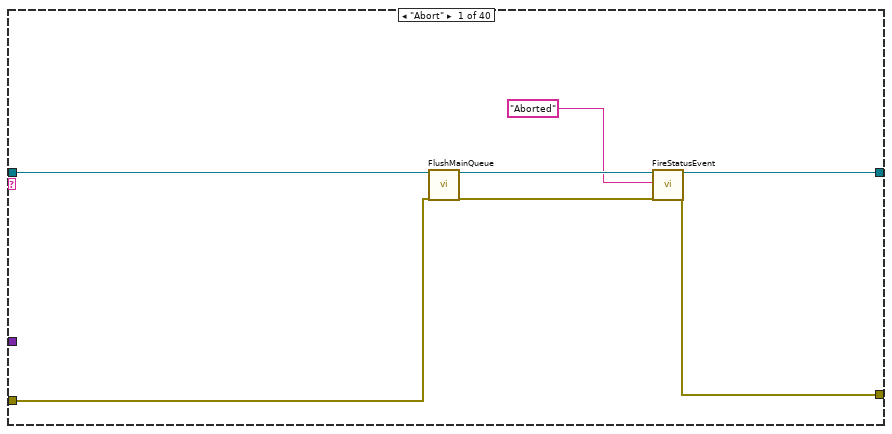
[diagram p2: hidden frame]
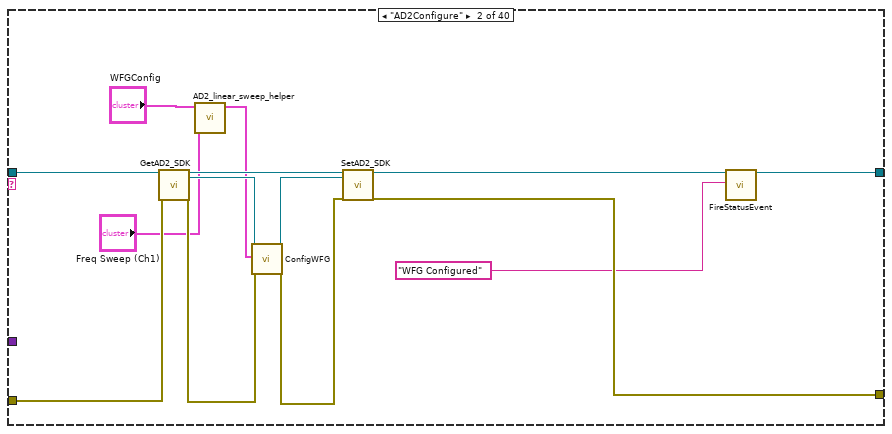
[diagram p3: hidden frame]
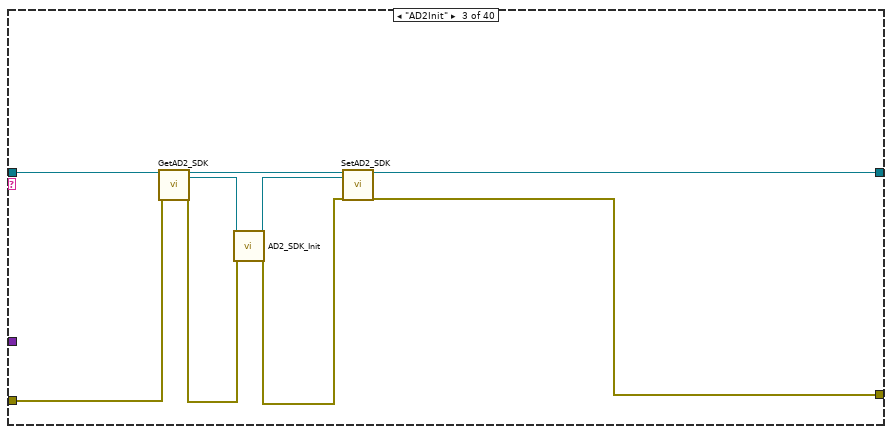
[diagram p4: hidden frame]
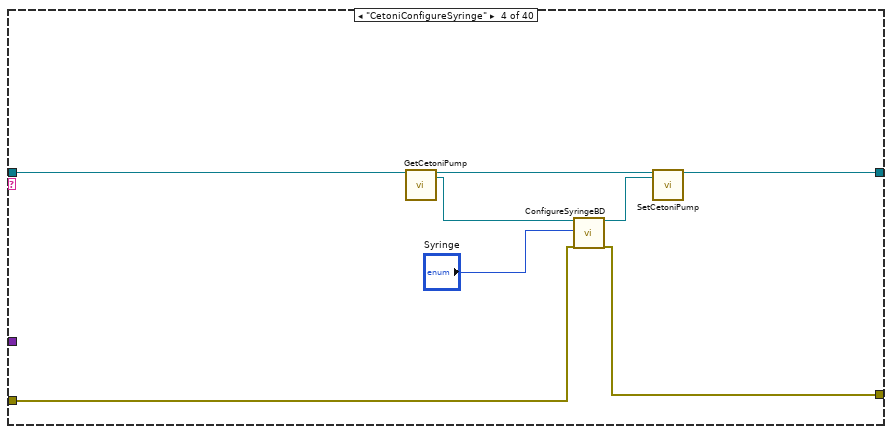
[diagram p5: hidden frame]
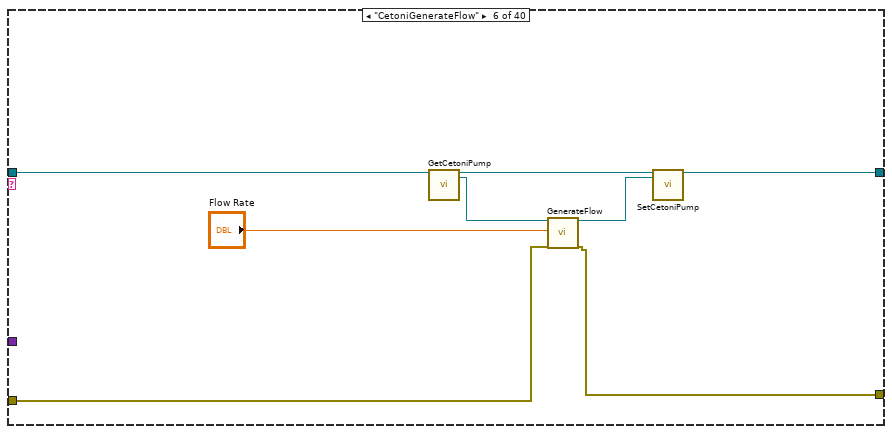
[diagram p6: hidden frame]
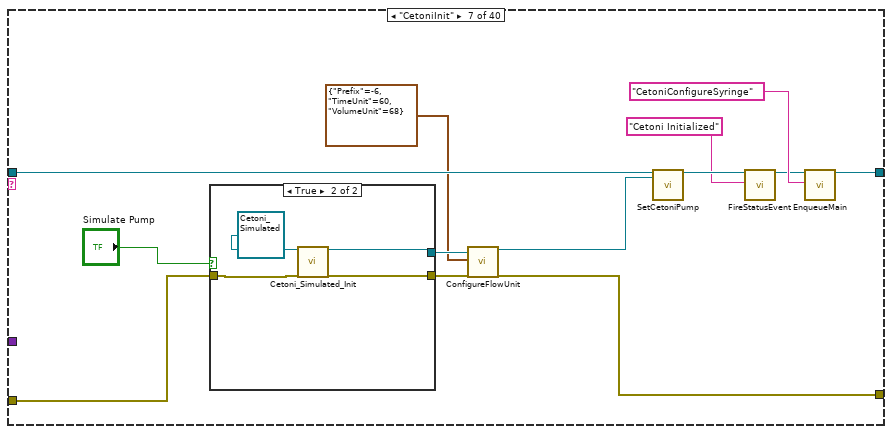
[diagram p7: hidden frame]
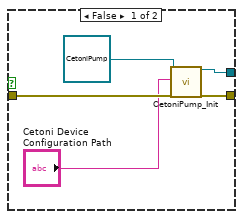
[diagram p8: hidden frame]
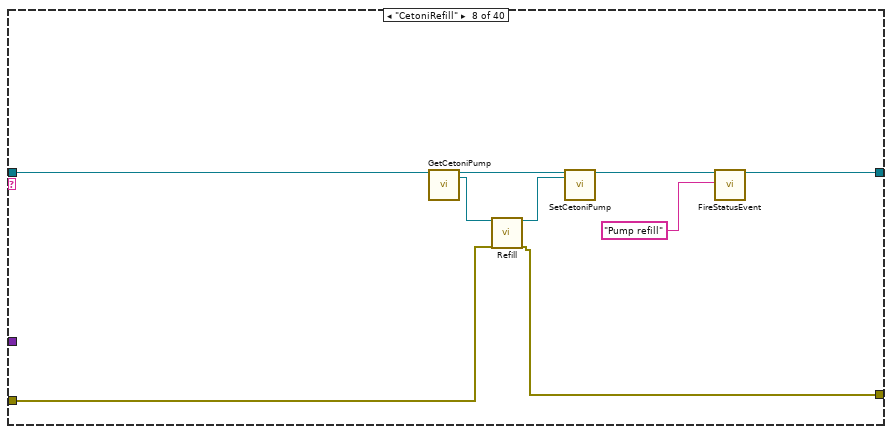
[diagram p9: hidden frame]
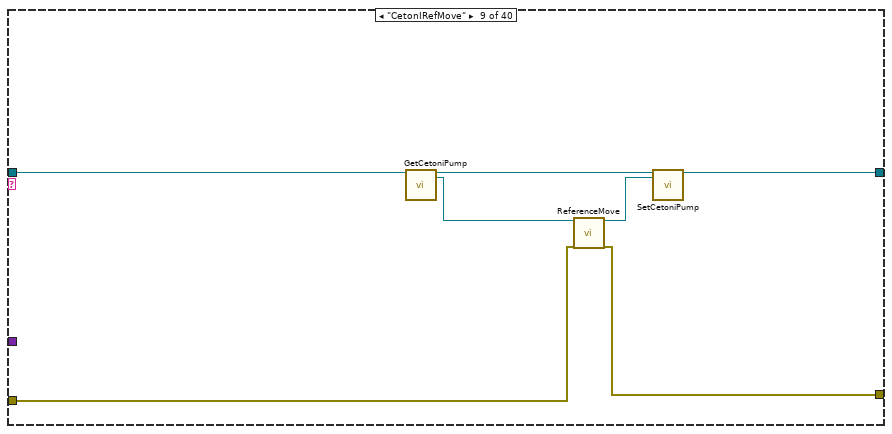
[diagram p10: hidden frame]
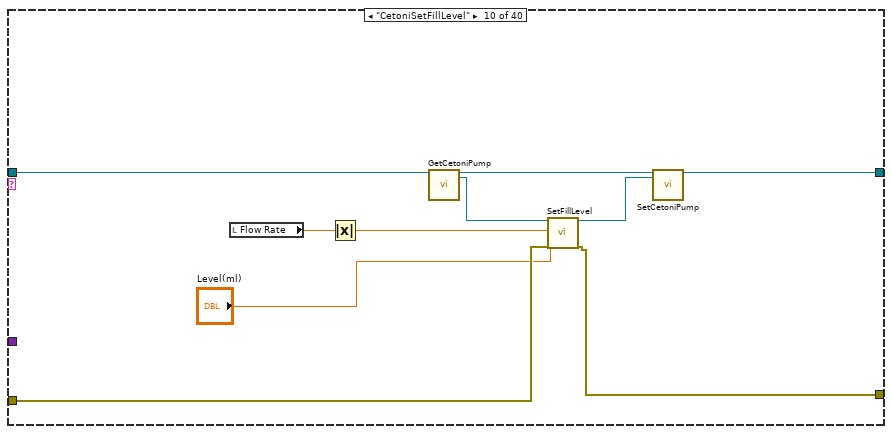
[diagram p11: hidden frame]
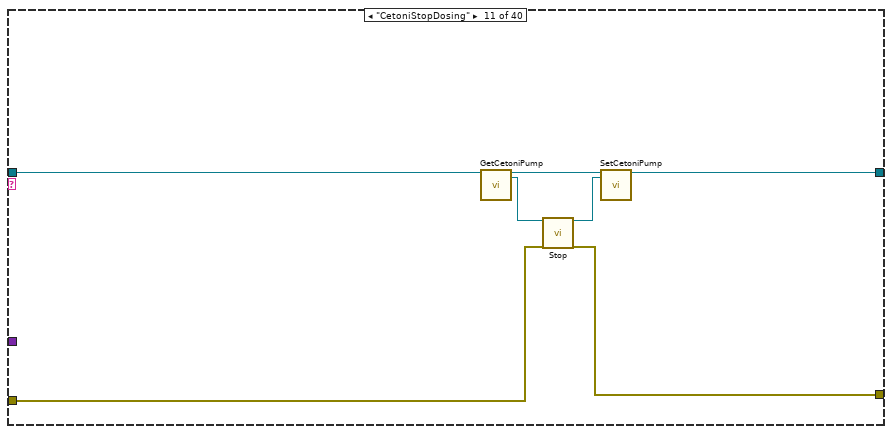
[diagram p12: hidden frame]
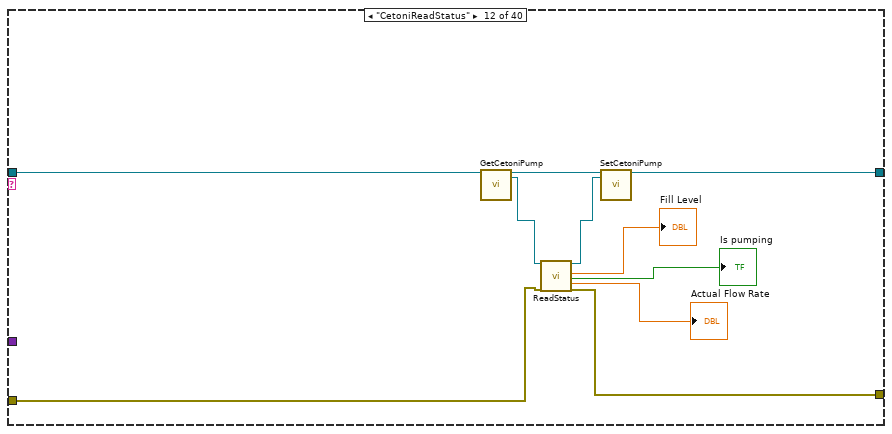
[diagram p13: hidden frame]
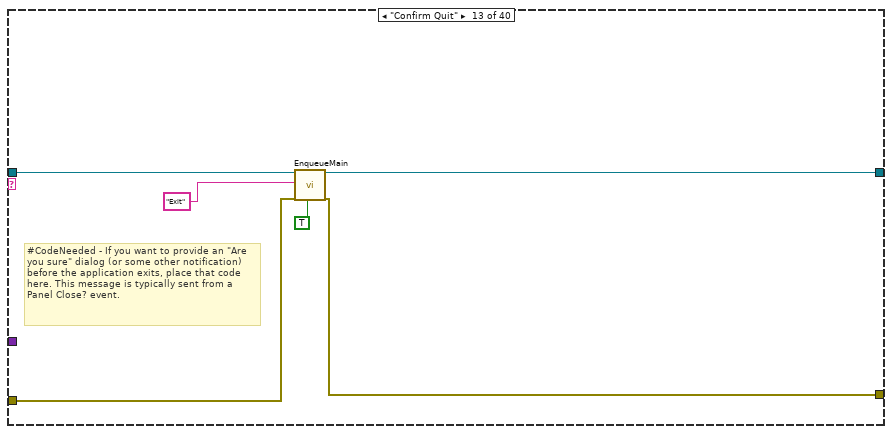
[diagram p14: hidden frame]
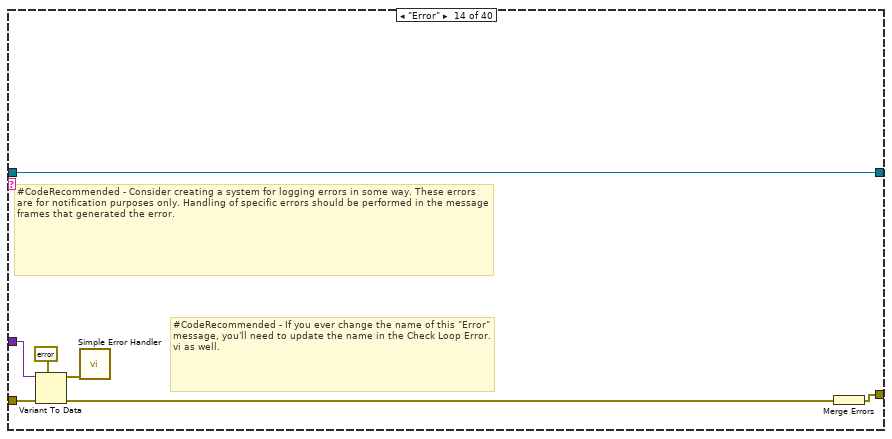
[diagram p15: hidden frame]
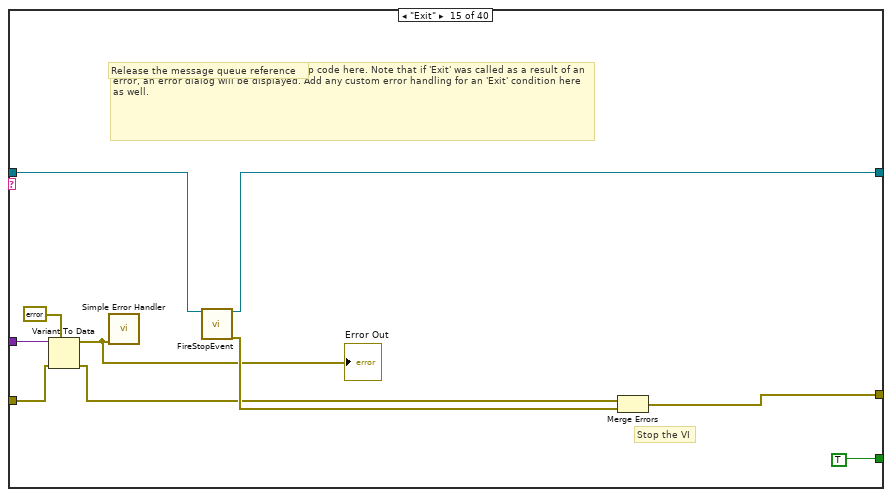
[diagram p16: hidden frame]
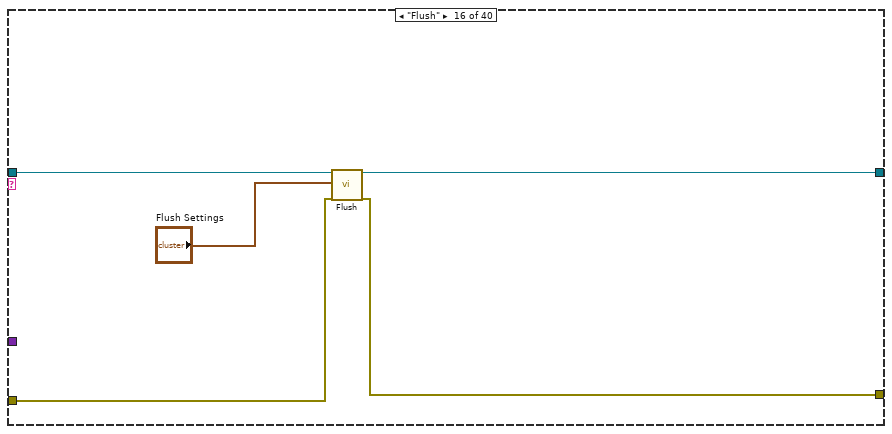
[diagram p17: hidden frame]
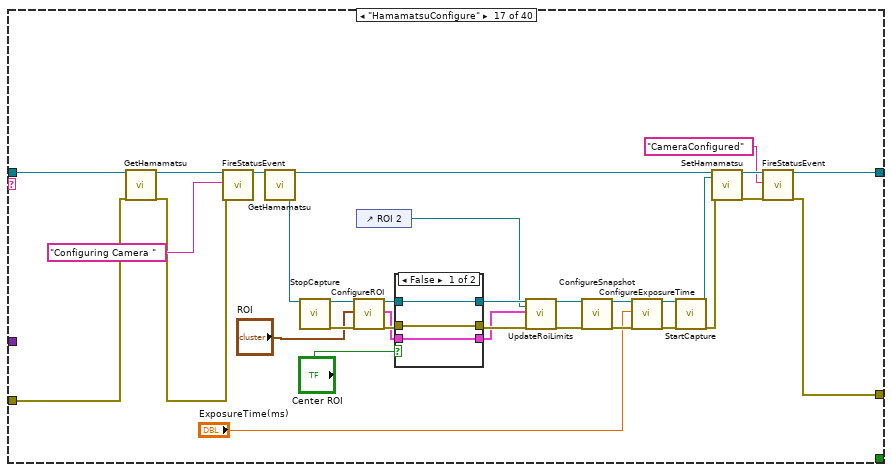
[diagram p18: hidden frame]
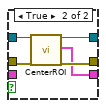
[diagram p19: hidden frame]
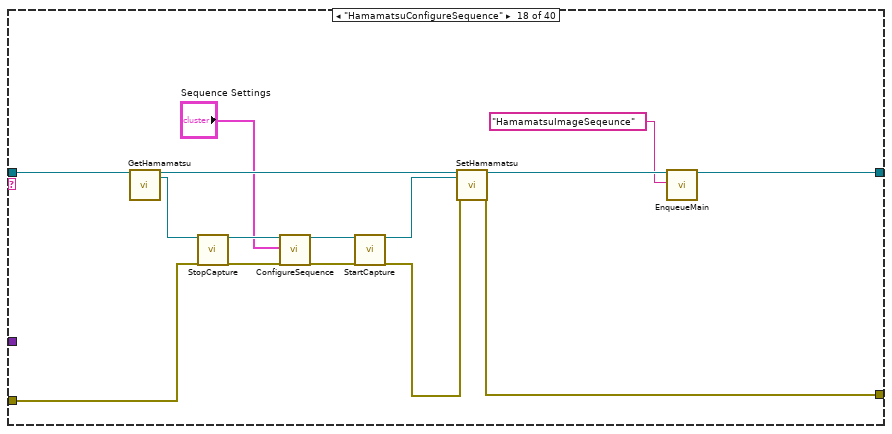
[diagram p20: hidden frame]
diagram:
  (unwired) "CetoniSetFillLevel" ("Message")
  (unwired) "CetoniGenerateFlow" ("Message")
  (unwired) "CetoniStopDosing" ("Message")
  (unwired) "CetoniEmpty" ("Message")
  (unwired) "CetoniRefill" ("Message")
  (unwired) "CetoniConfigureSyringe" ("Message")
  (unwired) "PumpInit" ("Message")
  n1 = call "Application_Init.vi"("object in"=refnum<class "Application.lvclass"> refnum ("Application")) -> ("object out"=w1:refnum<class "Application.lvclass">, "error out"=w8:errorcluster)  [unwired: 17 in]
  n2 = call-dynamic "RegisterEvents.vi"("object in"=w1, "error in (no error)"=w8) -> ("object out"=w9:refnum<class "Application.lvclass">, "Event Registration Refnum"=w10:refnum<event-registration>, "error out"=w2:errorcluster)  [unwired: 15 in]
  n3 = call-dynamic "FireStatusEvent.vi"("object in"=w1, "Status"="System Not Initialized", "error in (no error)"=w2) -> ()  [unwired: 15 in, 2 out]
  n4 = while {
    tunnel: w8 -> [w13]
    tunnel: [w17] -> w6
    shift-right: [w16] -> w5
    shift-left: w1 -> [w21]
    stop <- w22 stop-if-true
    # "Message Handling Loop"
    n5 = call-dynamic "DeQueueMain.vi"("object in"=w21, "error in (no error)"=w13) -> ("object out"=w12:refnum<class "Application.lvclass">, "Message"=w20:string, "Message Data"=w19:variant, "error out"=w14:errorcluster)  [unwired: 13 in, 1 out]
    n6 = case "Message Cases" shown="\"CetoniEmpty\"" w20 {
      selector: w20 -> [_ _ _ _ _ _ _ _ _ _ _ _ _ _ _ _ _ _ _ _ _ _ _ _ _ _ _ _ _ _ _ _ _ _ _ _ _ _ _ w558]
      tunnel: w14 -> [w27 w40 w47 w56 w64 w71 w88 w103 w111 w119 w126 w138 w148 w155 w157 w168 w202 w221 w230 w261 w269 w304 w316 w334 w345 w358 w361 w376 w397 w411 w422 w444 w487 w494 w500 w520 w531 w537 w555 _]
      tunnel: [w24 w39 w45 w54 w65 w72 w82 w104 w109 w120 w127 w136 w147 w150 w164 w167 w175 w219 w227 w256 w270 w305 w314 w333 w354 w358 w364 w377 w391 w412 w434 w451 w488 w494 w501 w521 w532 w542 w554 w559] -> w18
      tunnel: [_ _ _ _ _ _ _ _ _ _ _ _ _ _ TRUE _ _ _ _ _ _ _ _ _ _ _ _ _ _ _ _ _ _ _ _ _ _ _ _ _] -> w22
      tunnel: w19 -> [_ _ _ _ _ _ _ _ _ _ _ _ _ w154 w160 _ _ _ _ _ _ _ _ _ _ _ w363 _ _ _ _ _ _ _ _ _ _ w540 _ _]
      tunnel: w12 -> [w29 w43 w52 w60 w69 w77 w90 w108 w115 w125 w132 w142 w144 w149 w162 w170 w203 w226 w232 w266 w273 w312 w326 w341 w356 w357 w365 w372 w398 w413 w423 w446 w491 w495 w502 w522 w533 w549 w556 w557]
      tunnel: [w26 w34 w50 w58 w61 w75 w78 w100 w113 w123 w130 w140 w145 w149 w163 w169 w176 w218 w231 w264 w272 w311 w325 w340 w355 w357 w366 w383 w388 w414 w437 w450 w486 w493 w498 w515 w526 w544 w553 w557] -> w15
      frame "Abort" {
        n7 = call-dynamic "FlushMainQueue.vi"("object in"=w29, "error in (no error)"=w27) -> ("object out"=w28:refnum<class "Application.lvclass">, "error out"=w25:errorcluster)  [unwired: 15 in, 1 out]
        n8 = call-dynamic "FireStatusEvent.vi"("object in"=w28, "Status"="Aborted", "error in (no error)"=w25) -> ("object out"=w26:refnum<class "Application.lvclass">, "error out"=w24:errorcluster)  [unwired: 15 in]
      }
      frame "AD2Configure" {
        n9 = call-dynamic "GetAD2_SDK.vi"("object in"=w43, "error in (no error)"=w40) -> ("object out"=w42:refnum<class "Application.lvclass">, "AD2_SDK"=w38:refnum<class "AD2_SDK.lvclass">, "error out"=w36:errorcluster)  [unwired: 15 in]
        n10 = call "AD2_linear_sweep_helper.vi"("Freq Sweep (Ch1)"="Freq Sweep (Ch1)", "WFGConfig"="WFGConfig") -> ("WFGConfig 2"=w31:T2)  [unwired: 9 in]
        n11 = call-dynamic "ConfigWFG.vi"("object in"=w38, "Config(var)"=w31, "error in (no error)"=w36) -> ("object out"=w37:refnum<class "AD2_SDK.lvclass">, "error out"=w35:errorcluster)  [unwired: 15 in]
        n12 = call-dynamic "SetAD2_SDK.vi"("object in"=w42, "AD2_SDK"=w37, "error in (no error)"=w35) -> ("object out"=w41:refnum<class "Application.lvclass">, "error out"=w39:errorcluster)  [unwired: 15 in]
        n13 = call-dynamic "FireStatusEvent.vi"("object in"=w41, "Status"="WFG Configured") -> ("object out"=w34:refnum<class "Application.lvclass">)  [unwired: 16 in, 1 out]
      }
      frame "AD2Init" {
        n14 = call-dynamic "GetAD2_SDK.vi"("object in"=w52, "error in (no error)"=w47) -> ("object out"=w51:refnum<class "Application.lvclass">, "AD2_SDK"=w49:refnum<class "AD2_SDK.lvclass">, "error out"=w44:errorcluster)  [unwired: 15 in]
        n15 = call "AD2_SDK_Init.vi"("object in"=w49, "error in (no error)"=w44) -> ("object out"=w48:refnum<class "AD2_SDK.lvclass">, "error out"=w46:errorcluster)  [unwired: 16 in]
        n16 = call-dynamic "SetAD2_SDK.vi"("object in"=w51, "AD2_SDK"=w48, "error in (no error)"=w46) -> ("object out"=w50:refnum<class "Application.lvclass">, "error out"=w45:errorcluster)  [unwired: 15 in]
      }
      frame "CetoniConfigureSyringe" {
        n17 = call-dynamic "GetCetoniPump.vi"("object in"=w60) -> ("object out"=w59:refnum<class "Application.lvclass">, "CetoniPump"=w57:refnum<class "CetoniPump.lvclass">)  [unwired: 16 in, 1 out]
        n18 = call-dynamic "ConfigureSyringeBD.vi"("object in"=w57, "Syringe"="Syringe", "error in (no error)"=w56) -> ("object out"=w55:refnum<class "CetoniPump.lvclass">, "error out"=w54:errorcluster)  [unwired: 15 in]
        n19 = call-dynamic "SetCetoniPump.vi"("object in"=w59, "CetoniPump"=w55) -> ("object out"=w58:refnum<class "Application.lvclass">)  [unwired: 16 in, 1 out]
      }
      frame "CetoniEmpty" {
        n20 = call-dynamic "GetCetoniPump.vi"("object in"=w69) -> ("object out"=w68:refnum<class "Application.lvclass">, "CetoniPump"=w67:refnum<class "CetoniPump.lvclass">)  [unwired: 16 in, 1 out]
        n21 = call-dynamic "Empty.vi"("object in"=w67, "error in (no error)"=w64) -> ("object out"=w66:refnum<class "CetoniPump.lvclass">, "error out"=w65:errorcluster)  [unwired: 16 in]
        n22 = call-dynamic "SetCetoniPump.vi"("object in"=w68, "CetoniPump"=w66) -> ("object out"=w62:refnum<class "Application.lvclass">)  [unwired: 16 in, 1 out]
        n23 = call-dynamic "FireStatusEvent.vi"("object in"=w62, "Status"="Pump empty") -> ("object out"=w61:refnum<class "Application.lvclass">)  [unwired: 16 in, 1 out]
      }
      frame "CetoniGenerateFlow" {
        n24 = call-dynamic "GetCetoniPump.vi"("object in"=w77) -> ("object out"=w76:refnum<class "Application.lvclass">, "CetoniPump"=w74:refnum<class "CetoniPump.lvclass">)  [unwired: 16 in, 1 out]
        n25 = call-dynamic "GenerateFlow.vi"("object in"=w74, "Flow Rate"="Flow Rate", "error in (no error)"=w71) -> ("object out"=w73:refnum<class "CetoniPump.lvclass">, "error out"=w72:errorcluster)  [unwired: 15 in]
        n26 = call-dynamic "SetCetoniPump.vi"("object in"=w76, "CetoniPump"=w73) -> ("object out"=w75:refnum<class "Application.lvclass">)  [unwired: 16 in, 1 out]
      }
      frame "CetoniInit" {
        n27 = case shown="True" "Simulate Pump" {
          tunnel: [w95 w98] -> w89
          tunnel: w88 -> [w94 w97]
          tunnel: [w93 w96] -> w83
          frame False {
            n28 = call "CetoniPump_Init.vi"("object in"=refnum<class "CetoniPump.lvclass"> refnum, "Device Configuration Path"="Cetoni Device Configuration Path", "error in (no error)"=w94) -> ("object out"=w95:refnum<class "CetoniPump.lvclass">, "error out"=w93:errorcluster)  [unwired: 15 in]
          }
          frame True {
            n29 = call "Cetoni_Simulated_Init.vi"("object in"=refnum<class "Cetoni_Simulated.lvclass"> refnum ("Cetoni_Simulated"), "error in (no error)"=w97) -> ("object out"=w98:refnum<class "Cetoni_Simulated.lvclass">, "error out"=w96:errorcluster)  [unwired: 16 in]
          }
        }
        n30 = call-dynamic "ConfigureFlowUnit.vi"("object in"=w89, "SyringeSettings"=T21 {"Prefix"=-6, "TimeUnit"=60, "VolumeUnit"=68}, "error in (no error)"=w83) -> ("object out"=w85:refnum<class "CetoniPump.lvclass">, "error out"=w82:errorcluster)  [unwired: 15 in]
        n31 = call-dynamic "SetCetoniPump.vi"("object in"=w90, "CetoniPump"=w85) -> ("object out"=w87:refnum<class "Application.lvclass">)  [unwired: 16 in, 1 out]
        n32 = call-dynamic "FireStatusEvent.vi"("object in"=w87, "Status"="Cetoni Initialized") -> ("object out"=w79:refnum<class "Application.lvclass">)  [unwired: 16 in, 1 out]
        n33 = call-dynamic "EnqueueMain.vi"("object in"=w79, "Message"="CetoniConfigureSyringe") -> ("object out"=w78:refnum<class "Application.lvclass">)  [unwired: 16 in, 1 out]
      }
      frame "CetoniRefill" {
        n34 = call-dynamic "GetCetoniPump.vi"("object in"=w108) -> ("object out"=w107:refnum<class "Application.lvclass">, "CetoniPump"=w106:refnum<class "CetoniPump.lvclass">)  [unwired: 16 in, 1 out]
        n35 = call-dynamic "Refill.vi"("object in"=w106, "error in (no error)"=w103) -> ("object out"=w105:refnum<class "CetoniPump.lvclass">, "error out"=w104:errorcluster)  [unwired: 16 in]
        n36 = call-dynamic "SetCetoniPump.vi"("object in"=w107, "CetoniPump"=w105) -> ("object out"=w101:refnum<class "Application.lvclass">)  [unwired: 16 in, 1 out]
        n37 = call-dynamic "FireStatusEvent.vi"("object in"=w101, "Status"="Pump refill") -> ("object out"=w100:refnum<class "Application.lvclass">)  [unwired: 16 in, 1 out]
      }
      frame "CetonIRefMove" {
        n38 = call-dynamic "GetCetoniPump.vi"("object in"=w115) -> ("object out"=w114:refnum<class "Application.lvclass">, "CetoniPump"=w112:refnum<class "CetoniPump.lvclass">)  [unwired: 16 in, 1 out]
        n39 = call-dynamic "ReferenceMove.vi"("object in"=w112, "error in (no error)"=w111) -> ("object out"=w110:refnum<class "CetoniPump.lvclass">, "error out"=w109:errorcluster)  [unwired: 16 in]
        n40 = call-dynamic "SetCetoniPump.vi"("object in"=w114, "CetoniPump"=w110) -> ("object out"=w113:refnum<class "Application.lvclass">)  [unwired: 16 in, 1 out]
      }
      frame "CetoniSetFillLevel" {
        n41 = local read "Flow Rate"() -> (w117:dbl)
        n42 = Absolute Value(x=w117) -> (abs(x)=w116:dbl)
        n43 = call-dynamic "GetCetoniPump.vi"("object in"=w125) -> ("object out"=w124:refnum<class "Application.lvclass">, "CetoniPump"=w122:refnum<class "CetoniPump.lvclass">)  [unwired: 16 in, 1 out]
        n44 = call-dynamic "SetFillLevel.vi"("object in"=w122, "Flow"=w116, "Level(ml)"="Level(ml)", "error in (no error)"=w119) -> ("object out"=w121:refnum<class "CetoniPump.lvclass">, "error out"=w120:errorcluster)  [unwired: 14 in]
        n45 = call-dynamic "SetCetoniPump.vi"("object in"=w124, "CetoniPump"=w121) -> ("object out"=w123:refnum<class "Application.lvclass">)  [unwired: 16 in, 1 out]
      }
      frame "CetoniStopDosing" {
        n46 = call-dynamic "GetCetoniPump.vi"("object in"=w132) -> ("object out"=w131:refnum<class "Application.lvclass">, "CetoniPump"=w129:refnum<class "CetoniPump.lvclass">)  [unwired: 16 in, 1 out]
        n47 = call-dynamic "Stop.vi"("object in"=w129, "error in (no error)"=w126) -> ("object out"=w128:refnum<class "CetoniPump.lvclass">, "error out"=w127:errorcluster)  [unwired: 16 in]
        n48 = call-dynamic "SetCetoniPump.vi"("object in"=w131, "CetoniPump"=w128) -> ("object out"=w130:refnum<class "Application.lvclass">)  [unwired: 16 in, 1 out]
      }
      frame "CetoniReadStatus" {
        n49 = call-dynamic "GetCetoniPump.vi"("object in"=w142) -> ("object out"=w141:refnum<class "Application.lvclass">, "CetoniPump"=w139:refnum<class "CetoniPump.lvclass">)  [unwired: 16 in, 1 out]
        n50 = call-dynamic "ReadStatus.vi"("object in"=w139, "error in (no error)"=w138) -> ("object out"=w137:refnum<class "CetoniPump.lvclass">, "Fill Level"=→"Fill Level":dbl, "Is pumping"=→"Is pumping":bool, "Actual Flow Rate"=→"Actual Flow Rate":dbl, "error out"=w136:errorcluster)  [unwired: 13 in]
        n51 = call-dynamic "SetCetoniPump.vi"("object in"=w141, "CetoniPump"=w137) -> ("object out"=w140:refnum<class "Application.lvclass">)  [unwired: 16 in, 1 out]
      }
      frame "Confirm Quit" {
        # "#CodeNeeded - If you want to provide an \"Are you sure\" dialog (or some other notification) before the application exits, place that code here. This message is typically sent from a Panel Close? event."
        # "Confirm Quit - Message that can confirm whether or not the user wants to exit the application."
        n52 = call-dynamic "EnqueueMain.vi"("object in"=w144, "Message"="Exit", "error in (no error)"=w148, "Priority Message? (F)"=TRUE) -> ("object out"=w145:refnum<class "Application.lvclass">, "error out"=w147:errorcluster)  [unwired: 14 in]
      }
      frame "Error" {
        # "#CodeRecommended - If you ever change the name of this \"Error\" message, you'll need to update the name in the Check Loop Error.vi as well."
        # "#CodeRecommended - Consider creating a system for logging errors in some way. These errors are for notification purposes only. Handling of specific errors should be performed in the message frames that generated the error."
        # "Error - Display an error dialog. This message is sent by the \"Error Handler\" VIs at the end of other loops in this application."
        n53 = Variant To Data(error in=w155, type=errorcluster {"status"=FALSE, "code"=0, "source"=""} ("error constant"), Variant=w154) -> (data=w152:errorcluster, error out=w151:errorcluster)
        n54 = call <vilib>:"Simple Error Handler.vi"("error in (no error)"=w152) -> ()  [unwired: 4 in, 5 out]
        n55 = Merge Errors(w151) -> (w150:errorcluster)
      }
      frame "Exit" {
        # "Stop the VI"
        # "Release the message queue reference"
        # "#CodeNeeded - Add any required cleanup code here. Note that if 'Exit' was called as a result of an error, an error dialog will be displayed. Add any custom error handling for an 'Exit' condition here as well."
        # "Exit - Exit the application."
        n56 = Variant To Data(error in=w157, type=errorcluster {"status"=FALSE, "code"=0, "source"=""} ("error in (no error)"), Variant=w160) -> (data=w156:errorcluster, error out=w158:errorcluster)
        "Error Out" <- w156
        n57 = call <vilib>:"Simple Error Handler.vi"("error in (no error)"=w156) -> ()  [unwired: 4 in, 5 out]
        n58 = call-dynamic "FireStopEvent.vi"("object in"=w162) -> ("object out"=w163:refnum<class "Application.lvclass">, "error out"=w161:errorcluster)  [unwired: 17 in]
        n59 = Merge Errors(w158, w161) -> (w164:errorcluster)
      }
      frame "Flush" {
        n60 = call-dynamic "Flush.vi"("object in"=w170, "Flush Settings"="Flush Settings", "error in (no error)"=w168) -> ("object out"=w169:refnum<class "Application.lvclass">, "error out"=w167:errorcluster)  [unwired: 15 in]
      }
      frame "HamamatsuConfigure" {
        n61 = call-dynamic "GetHamamatsu.vi"("object in"=w203, "error in (no error)"=w202) -> ("object out"=w177:refnum<class "Application.lvclass">, "error out"=w173:errorcluster)  [unwired: 15 in, 1 out]
        n62 = call-dynamic "FireStatusEvent.vi"("object in"=w177, "Status"="Configuring Camera ", "error in (no error)"=w173) -> ("object out"=w199:refnum<class "Application.lvclass">)  [unwired: 15 in, 1 out]
        n63 = call-dynamic "GetHamamatsu.vi"("object in"=w199) -> ("object out"=w201:refnum<class "Application.lvclass">, "Hamamatsu"=w189:refnum<class "Hamamatsu.lvclass">)  [unwired: 16 in, 1 out]
        n64 = call-dynamic "StopCapture.vi"("object in"=w189) -> ("object out"=w188:refnum<class "Hamamatsu.lvclass">, "error out"=w187:errorcluster)  [unwired: 17 in]
        n65 = call-dynamic "ConfigureROI.vi"("object in"=w188, "Sub Region"="ROI", "error in (no error)"=w187) -> ("object out"=w186:refnum<class "Hamamatsu.lvclass">, "SubRegionLimits"=w184:T22, "error out"=w185:errorcluster)  [unwired: 14 in]
        n66 = control-ref of="ROI 2"() -> (w171:refnum<vi>)
        n67 = case shown="False" "Center ROI" {
          tunnel: w186 -> [w204 w211]
          tunnel: [w204 w210] -> w183
          tunnel: w185 -> [w205 w209]
          tunnel: [w205 w208] -> w181
          tunnel: w184 -> [w206 _]
          tunnel: [w206 w207] -> w179
          frame False {
          }
          frame True {
            n68 = call-dynamic "CenterROI.vi"("object in"=w211, "error in (no error)"=w209) -> ("object out"=w210:refnum<class "Hamamatsu.lvclass">, "Sub Region"=w207:T24, "error out"=w208:errorcluster)  [unwired: 15 in]
          }
        }
        n69 = call-dynamic "UpdateRoiLimits.vi"("object in"=w183, "reference to front panel item"=w171, "SubRegionLimits"=w179, "error in (no error)"=w181) -> ("object out"=w182:refnum<class "Hamamatsu.lvclass">, "error out"=w180:errorcluster)  [unwired: 14 in]
        n70 = call-dynamic "ConfigureSnapshot.vi"("object in"=w182, "error in (no error)"=w180) -> ("object out"=w195:refnum<class "Hamamatsu.lvclass">, "error out"=w196:errorcluster)  [unwired: 16 in]
        n71 = call-dynamic "ConfigureExposureTime.vi"("object in"=w195, "ExposureTime(ms)"="ExposureTime(ms)", "error in (no error)"=w196) -> ("object out"=w193:refnum<class "Hamamatsu.lvclass">, "error out"=w192:errorcluster)  [unwired: 15 in]
        n72 = call-dynamic "StartCapture.vi"("object in"=w193, "error in (no error)"=w192) -> ("object out"=w191:refnum<class "Hamamatsu.lvclass">, "error out"=w190:errorcluster)  [unwired: 16 in]
        n73 = call-dynamic "SetHamamatsu.vi"("object in"=w201, "Hamamatsu"=w191, "error in (no error)"=w190) -> ("object out"=w200:refnum<class "Application.lvclass">, "error out"=w174:errorcluster)  [unwired: 15 in]
        n74 = call-dynamic "FireStatusEvent.vi"("object in"=w200, "Status"="CameraConfigured", "error in (no error)"=w174) -> ("object out"=w176:refnum<class "Application.lvclass">, "error out"=w175:errorcluster)  [unwired: 15 in]
      }
      frame "HamamatsuConfigureSequence" {
        n75 = call-dynamic "GetHamamatsu.vi"("object in"=w226) -> ("object out"=w225:refnum<class "Application.lvclass">, "Hamamatsu"=w224:refnum<class "Hamamatsu.lvclass">)  [unwired: 16 in, 1 out]
        n76 = call-dynamic "StopCapture.vi"("object in"=w224, "error in (no error)"=w221) -> ("object out"=w216:refnum<class "Hamamatsu.lvclass">, "error out"=w215:errorcluster)  [unwired: 16 in]
        n77 = call-dynamic "ConfigureSequence.vi"("object in"=w216, "Sequence Settings"="Sequence Settings", "error in (no error)"=w215) -> ("object out"=w213:refnum<class "Hamamatsu.lvclass">, "error out"=w214:errorcluster)  [unwired: 15 in]
        n78 = call-dynamic "StartCapture.vi"("object in"=w213, "error in (no error)"=w214) -> ("object out"=w222:refnum<class "Hamamatsu.lvclass">, "error out"=w220:errorcluster)  [unwired: 16 in]
        n79 = call-dynamic "SetHamamatsu.vi"("object in"=w225, "Hamamatsu"=w222, "error in (no error)"=w220) -> ("object out"=w223:refnum<class "Application.lvclass">, "error out"=w219:errorcluster)  [unwired: 15 in]
        n80 = call-dynamic "EnqueueMain.vi"("object in"=w223, "Message"="HamamatsuImageSeqeunce") -> ("object out"=w218:refnum<class "Application.lvclass">)  [unwired: 16 in, 1 out]
      }
      frame "HamamatsuImage" {
        n81 = call-dynamic "FireStatusEvent.vi"("object in"=w232, "Status"="Imaging", "error in (no error)"=w230) -> ("object out"=w243:refnum<class "Application.lvclass">, "error out"=w238:errorcluster)  [unwired: 15 in]
        n82 = call-dynamic "GetHamamatsu.vi"("object in"=w243, "error in (no error)"=w238) -> ("object out"=w245:refnum<class "Application.lvclass">, "Hamamatsu"=w241:refnum<class "Hamamatsu.lvclass">, "error out"=w229:errorcluster)  [unwired: 15 in]
        n83 = call-dynamic "CaptureSnapshot.vi"("object in"=w241, "error in (no error)"=w229) -> ("object out"=w240:refnum<class "Hamamatsu.lvclass">, "FreeRunningImage"=w239:T25, "error out"=w228:errorcluster)  [unwired: 14 in, 1 out]
        n84 = call "IMAQ WindDraw"("Resize to Image Size? (Y)"=FALSE, "error in (no error)"=w228, "Image"=w239) -> ("error out"=w234:errorcluster)  [unwired: 7 in, 1 out]
        n85 = call "IMAQ WindZoom 2"("error in (no error)"=w234, "Zoom to Fit? (False)"=TRUE) -> ()  [unwired: 6 in, 4 out]
        n86 = call-dynamic "SetHamamatsu.vi"("object in"=w245, "Hamamatsu"=w240, "error in (no error)"=w234) -> ("object out"=w244:refnum<class "Application.lvclass">, "error out"=w227:errorcluster)  [unwired: 15 in]
        n87 = case shown="False" "Image Continous" {
          tunnel: w244 -> [w246 w249]
          tunnel: [w246 w248] -> w231
          tunnel: "HamamatsuImage" ("Message") -> [_ w247]
          frame False {
          }
          frame True {
            n88 = call-dynamic "EnqueueMain.vi"("object in"=w249, "Message"=w247) -> ("object out"=w248:refnum<class "Application.lvclass">)  [unwired: 16 in, 1 out]
          }
        }
      }
      frame "HamamatsuImageSeqeunce" {
        n89 = call-dynamic "GetHamamatsu.vi"("object in"=w266) -> ("object out"=w263:refnum<class "Application.lvclass">, "Hamamatsu"=w262:refnum<class "Hamamatsu.lvclass">)  [unwired: 16 in, 1 out]
        n90 = call-dynamic "ImageSequence.vi"("object in"=w262, "error in (no error)"=w261) -> ("object out"=w253:refnum<class "Hamamatsu.lvclass">, "Frame Index"=→"Frame Index 2":i32, "Frame Count"=w251:i32, "error out"=w260:errorcluster)  [unwired: 14 in]
        "Frame Count 2" <- w251
        n91 = call-dynamic "GetCameraBufferSize.vi"("object in"=w253) -> ("CameraBufferSize"=w250:i32)  [unwired: 16 in, 2 out]
        n92 = Greater Or Equal?(x=w251, y=w250) -> (x >= y?=w252:bool)
        n93 = call-dynamic "SetHamamatsu.vi"("object in"=w263, "Hamamatsu"=w253, "error in (no error)"=w260) -> ("object out"=w265:refnum<class "Application.lvclass">, "error out"=w257:errorcluster)  [unwired: 15 in]
        n94 = Select(t="HamamatsuShowSequence" ("Message"), s=w252, f="HamamatsuImageSeqeunce" ("Message")) -> (s? t:f=w258:string)
        n95 = call-dynamic "EnqueueMain.vi"("object in"=w265, "Message"=w258, "error in (no error)"=w257) -> ("object out"=w264:refnum<class "Application.lvclass">, "error out"=w256:errorcluster)  [unwired: 15 in]
      }
      frame "HamamatsuInit" {
        n96 = call-dynamic "FireStatusEvent.vi"("object in"=w273, "Status"="Init Camera ", "error in (no error)"=w269) -> ("object out"=w292:refnum<class "Application.lvclass">, "error out"=w268:errorcluster)  [unwired: 15 in]
        n97 = case shown="True" "Simulate Camera" {
          tunnel: [w298 w302] -> w294
          tunnel: [w297 w301] -> w289
          tunnel: w268 -> [w296 w299]
          frame False {
            n98 = call "Hamamatsu_Init.vi"("object in"=refnum<class "Hamamatsu.lvclass"> refnum, "error in (no error)"=w296) -> ("object out"=w298:refnum<class "Hamamatsu.lvclass">, "error out"=w297:errorcluster)  [unwired: 16 in]
          }
          frame True {
            n99 = call "Hamamatsu_simulated_Init.vi"("object in"=refnum<class "Hamamatsu_simulated.lvclass"> refnum ("Hamamatsu_simulated"), "error in (no error)"=w299) -> ("object out"=w302:refnum<class "Hamamatsu_simulated.lvclass">, "error out"=w301:errorcluster)  [unwired: 16 in]
          }
        }
        n100 = call-dynamic "OpenCamera.vi"("object in"=w294, "error in (no error)"=w289) -> ("object out"=w281:refnum<class "Hamamatsu.lvclass">, "error out"=w275:errorcluster)  [unwired: 15 in, 1 out]
        n101 = control-ref of="ROI 2"() -> (w279:refnum<vi>)
        n102 = call-dynamic "ReadSubregionLimitsandValue.vi"("object in"=w281, "error in (no error)"=w275) -> ("object out"=w278:refnum<class "Hamamatsu.lvclass">, "Sub Region"=w280:T24, "error out"=w274:errorcluster)  [unwired: 15 in]
        n103 = call-dynamic "UpdateRoiLimits.vi"("object in"=w278, "reference to front panel item"=w279, "SubRegionLimits"=w280, "error in (no error)"=w274) -> ("object out"=w277:refnum<class "Hamamatsu.lvclass">, "error out"=w276:errorcluster)  [unwired: 14 in]
        n104 = call-dynamic "ConfigureSnapshot.vi"("object in"=w277, "error in (no error)"=w276) -> ("object out"=w287:refnum<class "Hamamatsu.lvclass">, "error out"=w288:errorcluster)  [unwired: 16 in]
        n105 = call-dynamic "ConfigureExposureTime.vi"("object in"=w287, "ExposureTime(ms)"=50.0, "error in (no error)"=w288) -> ("object out"=w285:refnum<class "Hamamatsu.lvclass">, "error out"=w284:errorcluster)  [unwired: 15 in]
        n106 = call-dynamic "StartCapture.vi"("object in"=w285, "error in (no error)"=w284) -> ("object out"=w283:refnum<class "Hamamatsu.lvclass">, "error out"=w282:errorcluster)  [unwired: 16 in]
        n107 = call-dynamic "SetHamamatsu.vi"("object in"=w292, "Hamamatsu"=w283, "error in (no error)"=w282) -> ("object out"=w293:refnum<class "Application.lvclass">, "error out"=w271:errorcluster)  [unwired: 15 in]
        n108 = call-dynamic "FireStatusEvent.vi"("object in"=w293, "Status"="Camera Initialized", "error in (no error)"=w271) -> ("object out"=w272:refnum<class "Application.lvclass">, "error out"=w270:errorcluster)  [unwired: 15 in]
      }
      frame "HamamatsuSaveSequence" {
        n109 = call-dynamic "FireStatusEvent.vi"("object in"=w312, "Status"="Saving Sequence") -> ("object out"=w309:refnum<class "Application.lvclass">)  [unwired: 16 in, 1 out]
        n110 = call-dynamic "GetHamamatsu.vi"("object in"=w309) -> ("object out"=w308:refnum<class "Application.lvclass">, "Hamamatsu"=w307:refnum<class "Hamamatsu.lvclass">)  [unwired: 16 in, 1 out]
        n111 = call-dynamic "saveSequence.vi"("object in"=w307, "folder path"="Sequence path", "error in (no error)"=w304) -> ("error out"=w305:errorcluster)  [unwired: 13 in, 3 out]
        n112 = call-dynamic "FireStatusEvent.vi"("object in"=w308, "Status"="Sequence Saved!") -> ("object out"=w311:refnum<class "Application.lvclass">)  [unwired: 16 in, 1 out]
      }
      frame "AD2ConfigureDO" {
        n113 = call-dynamic "FireStatusEvent.vi"("object in"=w326, "Status"="Configuring DO") -> ("object out"=w323:refnum<class "Application.lvclass">)  [unwired: 16 in, 1 out]
        n114 = call-dynamic "GetAD2_SDK.vi"("object in"=w323, "error in (no error)"=w316) -> ("object out"=w321:refnum<class "Application.lvclass">, "AD2_SDK"=w319:refnum<class "AD2_SDK.lvclass">, "error out"=w317:errorcluster)  [unwired: 15 in]
        n115 = call-dynamic "ConfigDOCustom.vi"("object in"=w319, 2:"?", "error in (no error)"=w317) -> ("object out"=w318:refnum<class "AD2_SDK.lvclass">, "error out"=w315:errorcluster)  [unwired: 15 in]
        n116 = call-dynamic "SetAD2_SDK.vi"("object in"=w321, "AD2_SDK"=w318, "error in (no error)"=w315) -> ("object out"=w320:refnum<class "Application.lvclass">, "error out"=w314:errorcluster)  [unwired: 15 in]
        n117 = call-dynamic "FireStatusEvent.vi"("object in"=w320, "Status"="Do Configured") -> ("object out"=w325:refnum<class "Application.lvclass">)  [unwired: 16 in, 1 out]
      }
      frame "AD2ConfigureDOClock" {
        n118 = call-dynamic "FireStatusEvent.vi"("object in"=w341, "Status"="Configuring DO") -> ("object out"=w338:refnum<class "Application.lvclass">)  [unwired: 16 in, 1 out]
        n119 = call-dynamic "GetAD2_SDK.vi"("object in"=w338, "error in (no error)"=w334) -> ("object out"=w336:refnum<class "Application.lvclass">, "AD2_SDK"=w332:refnum<class "AD2_SDK.lvclass">, "error out"=w330:errorcluster)  [unwired: 15 in]
        n120 = call-dynamic "ConfigDOClockSpezial.vi"("object in"=w332, "DO Trigger"="DO Trigger", "ClockSettings"="ClockSettings", "error in (no error)"=w330) -> ("object out"=w331:refnum<class "AD2_SDK.lvclass">, "error out"=w329:errorcluster)  [unwired: 14 in]
        n121 = call-dynamic "SetAD2_SDK.vi"("object in"=w336, "AD2_SDK"=w331, "error in (no error)"=w329) -> ("object out"=w335:refnum<class "Application.lvclass">, "error out"=w333:errorcluster)  [unwired: 15 in]
        n122 = call-dynamic "FireStatusEvent.vi"("object in"=w335, "Status"="Do Configured") -> ("object out"=w340:refnum<class "Application.lvclass">)  [unwired: 16 in, 1 out]
      }
      frame "HamamatsuShowSequence" {
        n123 = call-dynamic "GetHamamatsu.vi"("object in"=w356) -> ("object out"=w353:refnum<class "Application.lvclass">, "Hamamatsu"=w349:refnum<class "Hamamatsu.lvclass">)  [unwired: 16 in, 1 out]
        n124 = call "hamamatsushowseq.vi"("Enum"=enum16{"Get Path", "RunAsync"}."Get Path") -> ("path"=w351:path)  [unwired: 10 in]
        n125 = call-dynamic "GetHandleOut.vi"("object in"=w349) -> ("Handle out"=w347:u32)  [unwired: 16 in, 2 out]
        n126 = Open VI Reference(type specifier VI Refnum (for type only)=refnum<vi> refnum, vi path=w351, options=128) -> (vi reference=w348:refnum<vi>)  [unwired: 3 in, 1 out]
        n127 = call-by-ref "Start Asynchronous Call"(reference=w348, error in=w345, "Enum"=enum16{"Get Path", "RunAsync"}."RunAsync", "Handle in"=w347) -> (reference out=w343:refnum<vi>, error out=w342:errorcluster)  [unwired: 9 in, 1 out]
        n128 = call-dynamic "SetHamamatsu.vi"("object in"=w353, "Hamamatsu"=w349, "error in (no error)"=w345) -> ("object out"=w355:refnum<class "Application.lvclass">, "error out"=w354:errorcluster)  [unwired: 15 in]
        n129 = Close Reference(reference=w343, error in (no error)=w342) -> ()  [unwired: 1 out]
      }
      frame "Initialize" {
        # "Initialize - All initialization work should take place in this message, since other loops can potentially enqueue messages that execute immediately after this one."
      }
      frame "PriorGoToPos" {
        n130 = Variant To Data(error in=w361, type=0 ("Pos (um)"), Variant=w363) -> (data=w359:i32, error out=w362:errorcluster)
        n131 = call-dynamic "GetPrior_Zmotor.vi"("object in"=w365, "error in (no error)"=w362) -> ("object out"=w371:refnum<class "Application.lvclass">, "Prior_Zmotor"=w370:refnum<class "Prior_Zmotor.lvclass">, "error out"=w368:errorcluster)  [unwired: 15 in]
        n132 = call-dynamic "GoToAbsPos.vi"("object in"=w370, "Pos (um)"=w359, "error in (no error)"=w368) -> ("object out"=w369:refnum<class "Prior_Zmotor.lvclass">, "error out"=w367:errorcluster)  [unwired: 14 in, 1 out]
        n133 = call-dynamic "SetPrior_Zmotor.vi"("object in"=w371, "Prior_Zmotor"=w369, "error in (no error)"=w367) -> ("object out"=w366:refnum<class "Application.lvclass">, "error out"=w364:errorcluster)  [unwired: 15 in]
      }
      frame "PriorInit" {
        n134 = call-dynamic "FireStatusEvent.vi"("object in"=w372, "Status"="Initializing Prior Stage") -> ("object out"=w373:refnum<class "Application.lvclass">)  [unwired: 16 in, 1 out]
        n135 = call-dynamic "GetPrior_Zmotor.vi"("object in"=w373, "error in (no error)"=w376) -> ("object out"=w382:refnum<class "Application.lvclass">, "Prior_Zmotor"=w381:refnum<class "Prior_Zmotor.lvclass">, "error out"=w379:errorcluster)  [unwired: 15 in]
        n136 = call "Prior_Zmotor_Init.vi"("object in"=w381, "VISA resource name"="Prior Visa resource name", "error in (no error)"=w379) -> ("object out"=w380:refnum<class "Prior_Zmotor.lvclass">, "error out"=w378:errorcluster)  [unwired: 15 in]
        n137 = call-dynamic "SetPrior_Zmotor.vi"("object in"=w382, "Prior_Zmotor"=w380, "error in (no error)"=w378) -> ("object out"=w383:refnum<class "Application.lvclass">, "error out"=w377:errorcluster)  [unwired: 15 in]
      }
      frame "PriorReadPos" {
        n138 = call-dynamic "GetPrior_Zmotor.vi"("object in"=w398, "error in (no error)"=w397) -> ("object out"=w403:refnum<class "Application.lvclass">, "Prior_Zmotor"=w402:refnum<class "Prior_Zmotor.lvclass">, "error out"=w400:errorcluster)  [unwired: 15 in]
        n139 = call-dynamic "ReadPosition.vi"("object in"=w402, "error in (no error)"=w400) -> ("object out"=w401:refnum<class "Prior_Zmotor.lvclass">, "Position (um)"=w386:dbl, "error out"=w395:errorcluster)  [unwired: 15 in]
        "Position (um)" <- w386
        n140 = call-dynamic "readmovement.vi"("object in"=w401, "error in (no error)"=w395) -> ("object out"=w396:refnum<class "Prior_Zmotor.lvclass">, "IsMoving?"=w385:bool, "error out"=w389:errorcluster)  [unwired: 15 in]
        n141 = call-dynamic "SetPrior_Zmotor.vi"("object in"=w403, "Prior_Zmotor"=w396, "error in (no error)"=w389) -> ("object out"=w399:refnum<class "Application.lvclass">, "error out"=w392:errorcluster)  [unwired: 15 in]
        n142 = case shown="False" "Read Position" {
          tunnel: w399 -> [w405 w410]
          tunnel: [w405 w409] -> w394
          tunnel: "PriorReadPos" -> [_ w408]
          tunnel: w392 -> [w404 w407]
          tunnel: [w404 w406] -> w391
          frame False {
          }
          frame True {
            n143 = call-dynamic "EnqueueMain.vi"("object in"=w410, "Message"=w408, "error in (no error)"=w407) -> ("object out"=w409:refnum<class "Application.lvclass">, "error out"=w406:errorcluster)  [unwired: 15 in]
          }
        }
        n144 = Bundle("Position (um)"=w386, "IsMoving?"=w385) -> (w384:cluster{"Position (um)":dbl, "IsMoving?":bool})  [unwired: 1 in]
        n145 = call-dynamic "FireUIEvent.vi"("object in"=w394, "Message"="UpdatePrior", "Message Data"=w384) -> ("object out"=w388:refnum<class "Application.lvclass">)  [unwired: 15 in, 1 out]
      }
      frame "PriorZero" {
        n146 = call-dynamic "GetPrior_Zmotor.vi"("object in"=w413, "error in (no error)"=w411) -> ("object out"=w419:refnum<class "Application.lvclass">, "Prior_Zmotor"=w418:refnum<class "Prior_Zmotor.lvclass">, "error out"=w416:errorcluster)  [unwired: 15 in]
        n147 = call-dynamic "ZeroPos.vi"("object in"=w418, "error in (no error)"=w416) -> ("object out"=w417:refnum<class "Prior_Zmotor.lvclass">, "error out"=w415:errorcluster)  [unwired: 16 in]
        n148 = call-dynamic "SetPrior_Zmotor.vi"("object in"=w419, "Prior_Zmotor"=w417, "error in (no error)"=w415) -> ("object out"=w414:refnum<class "Application.lvclass">, "error out"=w412:errorcluster)  [unwired: 15 in]
      }
      frame "RunExperiment2" {
        n149 = call-dynamic "GetExperimentSeriesGeneral.vi"("object in"=w423) -> ("ExperimentSeriesGeneral"=w424:refnum<class "ExperimentSeries2.lvclass">)  [unwired: 16 in, 2 out]
        n150 = call-dynamic "See Elements Left.vi"("object in"=w424, "error in (no error)"=w422) -> ("# elements in queue"=w431:i32, "Elapsed Time"=→"Elapsed Time":dbl, "Time Left"=→"Time Left":dbl, "error out"=w432:errorcluster)  [unwired: 13 in, 1 out]
        "# elements in queue" <- w431
        n151 = Number To Decimal String(number=w431) -> (decimal integer string=w430:string)  [unwired: 1 in]
        n152 = Concatenate Strings("Run..." ("Status"), w430, " left..." ("string")) -> (w428:string)
        n153 = call-dynamic "FireStatusEvent.vi"("object in"=w423, "Status"=w428) -> ("object out"=w436:refnum<class "Application.lvclass">)  [unwired: 16 in, 1 out]
        n154 = call-dynamic "RunExperiment2.vi"("object in"=w436, "error in (no error)"=w432) -> ("object out"=w435:refnum<class "Application.lvclass">, "Average FPS"=→"Average FPS":dbl, "Waveform Graph"=→"Waveform Graph":dbl[], "Finished"=w433:bool, "error out"=w434:errorcluster)  [unwired: 13 in]
        n155 = case shown="True" w433 {
          tunnel: w435 -> [w440 w442]
          tunnel: [w439 w443] -> w437
          frame False {
            n156 = call-dynamic "EnqueueMain.vi"("object in"=w440, "Message"="RunExperiment2") -> ("object out"=w439:refnum<class "Application.lvclass">)  [unwired: 16 in, 1 out]
          }
          frame True {
            n157 = call-dynamic "FireStatusEvent.vi"("object in"=w442, "Status"="Series Complete") -> ("object out"=w443:refnum<class "Application.lvclass">)  [unwired: 16 in, 1 out]
          }
        }
      }
      frame "StartExperimentSeries2" {
        n158 = call-dynamic "FlushMainQueue.vi"("object in"=w446, "error in (no error)"=w444) -> ("object out"=w447:refnum<class "Application.lvclass">, "error out"=w445:errorcluster)  [unwired: 15 in, 1 out]
        n159 = call <vilib>:"Check if File or Folder Exists.vi"("path"="SeriesPath 2") -> ("file or folder exists?"=w448:bool)  [unwired: 8 in, 2 out]
        n160 = case shown="False" w448 {
          tunnel: w447 -> [w471 w484]
          tunnel: w445 -> [w465 w483]
          tunnel: [w481 w483] -> w451
          tunnel: [w480 w484] -> w450
          tunnel: "SeriesPath 2" -> [w475 _]
          frame False {
            n161 = call "ExperimentSeries2_Init.vi"("object in"=refnum<class "ExperimentSeries2.lvclass"> refnum, "error in (no error)"=w465) -> ("object out"=w468:refnum<class "ExperimentSeries2.lvclass">, "error out"=w466:errorcluster)  [unwired: 16 in]
            n162 = call-dynamic "CreateExperiments.vi"("object in"=w468, "SeriesPath"=w475, "Analog Discovery Settings"="Analog Discovery Settings", "Dyamic Camera Start Time"="Dynamic Camera Start Time", "GlobalExposure"="GlobalExposure", "error in (no error)"=w466, "Frequency List"="Frequency List", "Frames"="Frames", "Repeats"="Repeats", "ExposureTime(ms)"="ExposureTime(ms) 2", "Dynamic Frequency"="Dynamic Frequency \n(or center freq)", "Flush Settings"="Flush Settings 2", "Freq Sweep (Ch1) 2"="Freq Sweep (Ch1) 2", "Camera Start Array(s)"="Camera Start Array(s)") -> ("object out"=w476:refnum<class "ExperimentSeries2.lvclass">, "Array"=w470:refnum<class "Experiment2.lvclass">[], "error out"=w473:errorcluster)  [unwired: 3 in]
            n163 = call-dynamic "EnqueExperiments.vi"("object in"=w476, "element"=w470, "error in (no error)"=w473) -> ("object out"=w474:refnum<class "ExperimentSeries2.lvclass">, "error out"=w472:errorcluster)  [unwired: 15 in]
            n164 = call-dynamic "SetExperimentSeriesGeneral.vi"("object in"=w471, "ExperimentSeriesGeneral"=w474, "error in (no error)"=w472) -> ("object out"=w462:refnum<class "Application.lvclass">, "error out"=w481:errorcluster)  [unwired: 15 in]
            n165 = call-dynamic "EnqueueMain.vi"("object in"=w462, "Message"="CetoniStopDosing") -> ("object out"=w461:refnum<class "Application.lvclass">)  [unwired: 16 in, 1 out]
            n166 = call-dynamic "EnqueueMain.vi"("object in"=w461, "Message"="Flush") -> ("object out"=w477:refnum<class "Application.lvclass">)  [unwired: 16 in, 1 out]
            n167 = call-dynamic "EnqueueMain.vi"("object in"=w477, "Message"="RunExperiment2") -> ("object out"=w480:refnum<class "Application.lvclass">)  [unwired: 16 in, 1 out]
          }
          frame True {
            n168 = One Button Dialog(message="Folder must be unique!") -> ()  [unwired: 1 in, 1 out]
          }
        }
      }
      frame "Trigg" {
        n169 = call-dynamic "GetHamamatsu.vi"("object in"=w491) -> ("object out"=w490:refnum<class "Application.lvclass">, "Hamamatsu"=w489:refnum<class "Hamamatsu.lvclass">)  [unwired: 16 in, 1 out]
        n170 = call-dynamic "SWTrigg.vi"("object in"=w489, "error in (no error)"=w487) -> ("error out"=w488:errorcluster)  [unwired: 16 in, 1 out]
        n171 = call-dynamic "GetAD2_SDK.vi"("object in"=w490) -> ("object out"=w486:refnum<class "Application.lvclass">, "AD2_SDK"=w485:refnum<class "AD2_SDK.lvclass">)  [unwired: 16 in, 1 out]
        n172 = call-dynamic "PCTrig.vi"("object in"=w485) -> ()  [unwired: 17 in, 2 out]
      }
      frame "AD2Trigg" {
        n173 = call-dynamic "GetAD2_SDK.vi"("object in"=w495) -> ("object out"=w493:refnum<class "Application.lvclass">, "AD2_SDK"=w492:refnum<class "AD2_SDK.lvclass">)  [unwired: 16 in, 1 out]
        n174 = call-dynamic "PCTrig.vi"("object in"=w492) -> ()  [unwired: 17 in, 2 out]
      }
      frame "ValveInit" {
        n175 = case shown="False" "Simulate Valve" {
          tunnel: [w509 w512] -> w504
          tunnel: w500 -> [w508 w510]
          tunnel: [w507 w511] -> w499
          frame False {
            n176 = call "Valve_Init.vi"("object in"=refnum<class "Valve.lvclass"> refnum, "VISA resource name"="Valve  VISA resource name", "error in (no error)"=w508) -> ("object out"=w509:refnum<class "Valve.lvclass">, "error out"=w507:errorcluster)  [unwired: 15 in]
          }
          frame True {
            n177 = call "Valve_Sim_Init.vi"("object in"=refnum<class "Valve_Sim.lvclass"> refnum, "error in (no error)"=w510) -> ("object out"=w512:refnum<class "Valve_Sim.lvclass">, "error out"=w511:errorcluster)  [unwired: 16 in]
          }
        }
        n178 = call-dynamic "SetValve.vi"("object in"=w502, "Valve"=w504, "error in (no error)"=w499) -> ("object out"=w503:refnum<class "Application.lvclass">, "error out"=w501:errorcluster)  [unwired: 15 in]
        n179 = call-dynamic "FireStatusEvent.vi"("object in"=w503, "Status"="Valve Initialized") -> ("object out"=w498:refnum<class "Application.lvclass">)  [unwired: 16 in, 1 out]
      }
      frame "ValvePos1" {
        n180 = call-dynamic "GetValve.vi"("object in"=w522, "error in (no error)"=w520) -> ("object out"=w524:refnum<class "Application.lvclass">, "Valve"=w519:refnum<class "Valve.lvclass">, "error out"=w517:errorcluster)  [unwired: 15 in]
        n181 = call-dynamic "ValvePos1.vi"("object in"=w519, "error in (no error)"=w517) -> ("object out"=w518:refnum<class "Valve.lvclass">, "error out"=w516:errorcluster)  [unwired: 16 in]
        n182 = call-dynamic "SetValve.vi"("object in"=w524, "Valve"=w518, "error in (no error)"=w516) -> ("object out"=w523:refnum<class "Application.lvclass">, "error out"=w521:errorcluster)  [unwired: 15 in]
        n183 = call-dynamic "FireStatusEvent.vi"("object in"=w523, "Status"="Valve Opened") -> ("object out"=w515:refnum<class "Application.lvclass">)  [unwired: 16 in, 1 out]
      }
      frame "ValvePos2" {
        n184 = call-dynamic "GetValve.vi"("object in"=w533, "error in (no error)"=w531) -> ("object out"=w535:refnum<class "Application.lvclass">, "Valve"=w530:refnum<class "Valve.lvclass">, "error out"=w528:errorcluster)  [unwired: 15 in]
        n185 = call-dynamic "ValvePos2.vi"("object in"=w530, "error in (no error)"=w528) -> ("object out"=w529:refnum<class "Valve.lvclass">, "error out"=w527:errorcluster)  [unwired: 16 in]
        n186 = call-dynamic "SetValve.vi"("object in"=w535, "Valve"=w529, "error in (no error)"=w527) -> ("object out"=w534:refnum<class "Application.lvclass">, "error out"=w532:errorcluster)  [unwired: 15 in]
        n187 = call-dynamic "FireStatusEvent.vi"("object in"=w534, "Status"="Valve Closed") -> ("object out"=w526:refnum<class "Application.lvclass">)  [unwired: 16 in, 1 out]
      }
      frame "Wait" {
        n188 = Variant To Data(error in=w537, type=0.0 ("Wait (s)"), Variant=w540) -> (data=w536:dbl, error out=w538:errorcluster)
        n189 = call-dynamic "FireStatusEvent.vi"("object in"=w549, "Status"="Waiting", "error in (no error)"=w538) -> ("object out"=w548:refnum<class "Application.lvclass">, "error out"=w547:errorcluster)  [unwired: 15 in]
        n190 = call-dynamic "Wait.vi"("object in"=w548, "Wait (s)"=w536, "error in (no error)"=w547) -> ("object out"=w545:refnum<class "Application.lvclass">, "error out"=w543:errorcluster)  [unwired: 15 in]
        n191 = call-dynamic "FireStatusEvent.vi"("object in"=w545, "Status"="Wait Completed", "error in (no error)"=w543) -> ("object out"=w544:refnum<class "Application.lvclass">, "error out"=w542:errorcluster)  [unwired: 15 in]
      }
      frame "Zstack" {
        n192 = call-dynamic "ZStack.vi"("object in"=w556, "Top"="Top", "Bottom"="Bottom", "Step Size"="Step Size", "error in (no error)"=w555) -> ("object out"=w553:refnum<class "Application.lvclass">, "error out"=w554:errorcluster)  [unwired: 13 in]
      }
      frame Default {
        # "'Default' case only runs if there is a message that isn't defined in any of the other cases.  Output a programming error."
        n193 = xnode "Error Ring"("parameter 0"=w558) -> ("error out"=w559:errorcluster)
      }
    }
    n194 = call-dynamic "ErrorHandlerMainLoop.vi"("object in"=w15, "error in (no error)"=w18) -> ("object out"=w16:refnum<class "Application.lvclass">, "error out"=w17:errorcluster)  [unwired: 16 in]
  }
  n195 = while {
    shift-right: [w574] -> _
    shift-left: w10 -> [w575]
    tunnel: [w569] -> w7
    shift-right: [w567] -> _
    shift-left: w9 -> [w572]
    tunnel: w2 -> [w571]
    stop <- w573 stop-if-true
    # "Event Handling Loop"
    n196 = event shown="[10] \"Read Pump Status\": Value Change" {
      selector: w575 -> [_ _ _ _ _ _ _ _ _ _ _ _ _ _ _ _ _ _ _ _ _ _ _ _ _ _ _ _ _ _ _ _ _ _ _ _]
      dyn-events: [_ _ _ _ _ _ _ _ _ _ _ _ _ _ _ _ _ _ _ _ _ _ _ _ _ _ _ _ _ _ _ _ _ _ _ _] -> w574
      timeout: _ -> [_ _ _ _ _ _ _ _ _ _ _ _ _ _ _ _ _ _ _ _ _ _ _ _ _ _ _ _ _ _ _ _ _ _ _ _]
      tunnel: [_ _ _ _ _ _ _ _ _ _ _ _ _ _ _ _ _ _ _ _ _ _ _ _ _ _ _ _ _ _ _ TRUE ("Discard?") _ _ _ _] -> w573
      tunnel: [w578 w583 w586 w592 w598 w603 w608 w611 w616 w622 w627 w632 w637 w647 w652 w657 w662 w667 w671 w676 w683 w688 w693 w698 w703 w707 w711 w716 w721 w738 w746 w750 w754 w767 w772 w777] -> w570
      tunnel: w572 -> [w577 w584 w590 w595 w600 w605 w610 w615 w617 w624 w629 w634 w639 w649 w654 w660 w665 w670 w674 w679 w680 w685 w690 w695 w700 w706 w708 w713 w718 w724 w749 w751 w757 w770 w775 w780]
      tunnel: [w576 w584 w589 w594 w599 w604 w609 w614 w618 w623 w628 w633 w638 w648 w653 w659 w664 w669 w674 w678 w684 w689 w694 w699 w704 w706 w712 w717 w722 w723 w748 w751 w757 w769 w774 w779] -> w568
      tunnel: w571 -> [w579 w583 w585 w591 w597 w602 w607 w611 w616 w621 w626 w631 w636 w646 w651 w656 w661 w666 w673 w675 w682 w687 w692 w697 w702 w707 w710 w715 w720 w738 w745 w750 w755 w766 w771 w778]
      event Panel Close? {
        # "Send the 'Confirm Quit' message if the user closes the panel of the VI. Discard the event so the 'Confirm Quit' message has a chance to run."
        n197 = event-data() -> ()  [unwired: 1 in, 1 out]
        n198 = call-dynamic "EnqueueMain.vi"("object in"=w577, "Message"="Confirm Quit", "error in (no error)"=w579, "Priority Message? (F)"=TRUE) -> ("object out"=w576:refnum<class "Application.lvclass">, "error out"=w578:errorcluster)  [unwired: 14 in]
        n199 = event-data("Discard?"=TRUE) -> ()  [unwired: 1 in, 1 out]
      }
      event Application Instance Close {
        # "#CodeRecommended - When a project closes, all VIs within that project are aborted and leave memory. However, any code placed in this event frame is guaranteed to run to completion, so add any cleanup code that absolutely must happen here."
        n200 = event-data() -> ()  [unwired: 1 in, 1 out]
      }
      event "Exit": Value Change {
        n201 = event-data() -> ()  [unwired: 1 in, 1 out]
        n202 = call-dynamic "EnqueueMain.vi"("object in"=w590, "Message"="Exit", "Message Data"=w585, "Priority Message? (F)"=TRUE) -> ("object out"=w589:refnum<class "Application.lvclass">, "error out"=w586:errorcluster)  [unwired: 14 in]
      }
      event "Valve Pos1": Value Change {
        n203 = event-data() -> ()  [unwired: 1 in, 2 out]
        n204 = call-dynamic "EnqueueMain.vi"("object in"=w595, "Message"="ValvePos1", "error in (no error)"=w591) -> ("object out"=w594:refnum<class "Application.lvclass">, "error out"=w592:errorcluster)  [unwired: 15 in]
      }
      event "Refill": Value Change {
        n205 = event-data() -> ()  [unwired: 1 in, 2 out]
        n206 = call-dynamic "EnqueueMain.vi"("object in"=w600, "Message"="CetoniRefill", "error in (no error)"=w597) -> ("object out"=w599:refnum<class "Application.lvclass">, "error out"=w598:errorcluster)  [unwired: 15 in]
      }
      event "Empty": Value Change {
        n207 = event-data() -> ()  [unwired: 1 in, 2 out]
        n208 = call-dynamic "EnqueueMain.vi"("object in"=w605, "Message"="CetoniEmpty", "error in (no error)"=w602) -> ("object out"=w604:refnum<class "Application.lvclass">, "error out"=w603:errorcluster)  [unwired: 15 in]
      }
      event "ConfigureSyringe": Value Change {
        n209 = event-data() -> ()  [unwired: 1 in, 2 out]
        n210 = call-dynamic "EnqueueMain.vi"("object in"=w610, "Message"="CetoniConfigureSyringe", "error in (no error)"=w607) -> ("object out"=w609:refnum<class "Application.lvclass">, "error out"=w608:errorcluster)  [unwired: 15 in]
      }
      event "GoToPosPrior": Value Change {
        n211 = event-data() -> ()  [unwired: 1 in, 2 out]
        n212 = call-dynamic "EnqueueMain.vi"("object in"=w615, "Message"="PriorGoToPos", "Message Data"="Pos (um)") -> ("object out"=w614:refnum<class "Application.lvclass">)  [unwired: 15 in, 1 out]
      }
      event "Read Position": Value Change {
        n213 = event-data() -> ()  [unwired: 1 in, 2 out]
        n214 = call-dynamic "EnqueueMain.vi"("object in"=w617, "Message"="PriorReadPos") -> ("object out"=w618:refnum<class "Application.lvclass">)  [unwired: 16 in, 1 out]
      }
      event "Reference move": Value Change {
        n215 = event-data() -> ()  [unwired: 1 in, 2 out]
        n216 = call-dynamic "EnqueueMain.vi"("object in"=w624, "Message"="CetonIRefMove", "error in (no error)"=w621) -> ("object out"=w623:refnum<class "Application.lvclass">, "error out"=w622:errorcluster)  [unwired: 15 in]
      }
      event "Read Pump Status": Value Change {
        n217 = event-data() -> ()  [unwired: 1 in, 2 out]
        n218 = call-dynamic "EnqueueMain.vi"("object in"=w629, "Message"="CetoniReadStatus", "error in (no error)"=w626) -> ("object out"=w628:refnum<class "Application.lvclass">, "error out"=w627:errorcluster)  [unwired: 15 in]
      }
      event "Stop Syringe": Value Change {
        n219 = event-data() -> ()  [unwired: 1 in, 2 out]
        n220 = call-dynamic "EnqueueMain.vi"("object in"=w634, "Message"="CetoniStopDosing", "error in (no error)"=w631) -> ("object out"=w633:refnum<class "Application.lvclass">, "error out"=w632:errorcluster)  [unwired: 15 in]
      }
      event "Flush": Value Change {
        n221 = event-data() -> ()  [unwired: 1 in, 2 out]
        n222 = for {
          N: "Number of flushes" -> [_]
          shift-right: [w643] -> w638
          shift-left: w639 -> [w644]
          shift-right: [w642] -> w637
          shift-left: w636 -> [w641]
          n223 = call-dynamic "EnqueueMain.vi"("object in"=w644, "Message"="Flush", "error in (no error)"=w641) -> ("object out"=w643:refnum<class "Application.lvclass">, "error out"=w642:errorcluster)  [unwired: 15 in]
        }
      }
      event "Generate Flow": Value Change {
        n224 = event-data() -> ()  [unwired: 1 in, 2 out]
        n225 = call-dynamic "EnqueueMain.vi"("object in"=w649, "Message"="CetoniGenerateFlow", "error in (no error)"=w646) -> ("object out"=w648:refnum<class "Application.lvclass">, "error out"=w647:errorcluster)  [unwired: 15 in]
      }
      event "Go to Level": Value Change {
        n226 = event-data() -> ()  [unwired: 1 in, 2 out]
        n227 = call-dynamic "EnqueueMain.vi"("object in"=w654, "Message"="CetoniSetFillLevel", "error in (no error)"=w651) -> ("object out"=w653:refnum<class "Application.lvclass">, "error out"=w652:errorcluster)  [unwired: 15 in]
      }
      event "Abort": Value Change {
        n228 = event-data() -> ()  [unwired: 1 in, 2 out]
        n229 = call-dynamic "EnqueueMain.vi"("object in"=w660, "Message"="Abort", "error in (no error)"=w656, "Priority Message? (F)"=TRUE) -> ("object out"=w659:refnum<class "Application.lvclass">, "error out"=w657:errorcluster)  [unwired: 14 in]
      }
      event "ValvePos2": Value Change {
        n230 = event-data() -> ()  [unwired: 1 in, 2 out]
        n231 = call-dynamic "EnqueueMain.vi"("object in"=w665, "Message"="ValvePos2", "error in (no error)"=w661) -> ("object out"=w664:refnum<class "Application.lvclass">, "error out"=w662:errorcluster)  [unwired: 15 in]
      }
      event "Configure Camera": Value Change {
        n232 = event-data() -> ()  [unwired: 1 in, 2 out]
        n233 = call-dynamic "EnqueueMain.vi"("object in"=w670, "Message"="HamamatsuConfigure", "error in (no error)"=w666) -> ("object out"=w669:refnum<class "Application.lvclass">, "error out"=w667:errorcluster)  [unwired: 15 in]
      }
      event "Frequency List Generator": Value Change {
        n234 = event-data() -> ()  [unwired: 1 in, 2 out]
        n235 = call "FrequencyHelper.vi"("error in (no error)"=w673) -> ("error out"=w671:errorcluster, "List of Frequencies (Hz)"=w672:dbl[])  [unwired: 9 in]
        n236 = local write "Frequency List"(w672) -> ()
      }
      event "Start Experiment series": Value Change {
        n237 = event-data() -> ()  [unwired: 1 in, 2 out]
        n238 = call-dynamic "EnqueueMain.vi"("object in"=w679, "Message"="StartExperimentSeries2", "error in (no error)"=w675) -> ("object out"=w678:refnum<class "Application.lvclass">, "error out"=w676:errorcluster)  [unwired: 15 in]
      }
      event "Image": Value Change {
        n239 = event-data() -> ()  [unwired: 1 in, 2 out]
        n240 = call-dynamic "EnqueueMain.vi"("object in"=w680, "Message"="HamamatsuImage", "error in (no error)"=w682) -> ("object out"=w684:refnum<class "Application.lvclass">, "error out"=w683:errorcluster)  [unwired: 15 in]
      }
      event "StartSequence": Value Change {
        n241 = event-data() -> ()  [unwired: 1 in, 2 out]
        n242 = call-dynamic "EnqueueMain.vi"("object in"=w685, "Message"="HamamatsuConfigureSequence", "error in (no error)"=w687) -> ("object out"=w689:refnum<class "Application.lvclass">, "error out"=w688:errorcluster)  [unwired: 15 in]
      }
      event "Configure DO": Value Change {
        n243 = event-data() -> ()  [unwired: 1 in, 2 out]
        n244 = call-dynamic "EnqueueMain.vi"("object in"=w690, "Message"="AD2ConfigureDO", "error in (no error)"=w692) -> ("object out"=w694:refnum<class "Application.lvclass">, "error out"=w693:errorcluster)  [unwired: 15 in]
      }
      event "Configure DO Clock": Value Change {
        n245 = event-data() -> ()  [unwired: 1 in, 2 out]
        n246 = call-dynamic "EnqueueMain.vi"("object in"=w695, "Message"="AD2ConfigureDOClock", "error in (no error)"=w697) -> ("object out"=w699:refnum<class "Application.lvclass">, "error out"=w698:errorcluster)  [unwired: 15 in]
      }
      event "TriggAD2": Value Change {
        n247 = event-data() -> ()  [unwired: 1 in, 2 out]
        n248 = call-dynamic "EnqueueMain.vi"("object in"=w700, "Message"="AD2Trigg", "error in (no error)"=w702) -> ("object out"=w704:refnum<class "Application.lvclass">, "error out"=w703:errorcluster)  [unwired: 15 in]
      }
      event "Adjust Intensity in image": Value Change {
        n249 = event-data() -> ()  [unwired: 1 in, 2 out]
        n250 = call "IMAQ WindDisplayMapping"("Conversion Policy (Default)"="Conversion Policy (Default)") -> ()  [unwired: 9 in, 2 out]
      }
      event "SaveSequence": Value Change {
        n251 = event-data() -> ()  [unwired: 1 in, 2 out]
        n252 = call-dynamic "EnqueueMain.vi"("object in"=w708, "Message"="HamamatsuSaveSequence", "error in (no error)"=w710) -> ("object out"=w712:refnum<class "Application.lvclass">, "error out"=w711:errorcluster)  [unwired: 15 in]
      }
      event "Trigg": Value Change {
        n253 = event-data() -> ()  [unwired: 1 in, 2 out]
        n254 = call-dynamic "EnqueueMain.vi"("object in"=w713, "Message"="Trigg", "error in (no error)"=w715) -> ("object out"=w717:refnum<class "Application.lvclass">, "error out"=w716:errorcluster)  [unwired: 15 in]
      }
      event "Flush": Value Change {
        n255 = event-data() -> ()  [unwired: 1 in, 2 out]
        n256 = call-dynamic "EnqueueMain.vi"("object in"=w718, "Message"="Flush", "error in (no error)"=w720) -> ("object out"=w722:refnum<class "Application.lvclass">, "error out"=w721:errorcluster)  [unwired: 15 in]
      }
      event "Initialize System": Value Change {
        n257 = event-data() -> ()  [unwired: 1 in, 2 out]
        n258 = Build Array("Z stage", "Analog Discovery 3", "Hamamatsu", "Cetoni Pump", "MX Valve 2") -> (w726:bool[])
        n259 = Build Array("PriorInit" ("Message"), "AD2Init" ("Message"), "HamamatsuInit" ("Message"), "CetoniInit" ("Message"), "ValveInit" ("Message")) -> (w727:string[])
        n260 = for {
          tunnel: w727 -> [w743] mode=indexing
          tunnel: w726 -> [w742] mode=indexing
          tunnel: [w743] -> w725 mode=indexing if=w742
        }
        n261 = for {
          tunnel: w725 -> [w740] mode=indexing
          shift-right: [w739] -> w723
          shift-left: w724 -> [w741]
          n262 = call-dynamic "EnqueueMain.vi"("object in"=w741, "Message"=w740) -> ("object out"=w739:refnum<class "Application.lvclass">)  [unwired: 16 in, 1 out]
        }
      }
      event "Send Pump Command": Value Change {
        n263 = event-data() -> ()  [unwired: 1 in, 2 out]
        n264 = call-dynamic "EnqueueMain.vi"("object in"=w749, "Message"="Pump", "Message Data"="Command", "error in (no error)"=w745) -> ("object out"=w748:refnum<class "Application.lvclass">, "error out"=w746:errorcluster)  [unwired: 14 in]
      }
      event User Event {
        (unwired) "\"Exit\" button pressed" ("VI Stopped")
        # "The Message Handling Loop processed an \"Exit\" message, which fired this event to stop the Event Handling Loop."
        n265 = event-data() -> ()  [unwired: 1 in, 1 out]
      }
      event User Event {
        n266 = event-data() -> ("Message"=w756:string, "Message Data"=w753:variant)  [unwired: 1 in, 4 out]
        n267 = case shown="\"UpdateStatus\"" w756 {
          tunnel: w755 -> [w758 w763]
          tunnel: [w759 w762] -> w754
          tunnel: w753 -> [_ w761]
          frame "False", Default {
            n268 = Merge Errors(errorcluster {"status"=TRUE, "code"=5005, "source"="INvalid String In Message Handling Loop"} ("error in (no error)"), w758) -> (w759:errorcluster)
          }
          frame "UpdateStatus" {
            n269 = Variant To Data(error in=w763, type="", Variant=w761) -> (data=→"Status":string, error out=w762:errorcluster)
          }
        }
      }
      event "Get Z Stack": Value Change {
        n270 = event-data() -> ()  [unwired: 1 in, 6 out]
        n271 = call-dynamic "EnqueueMain.vi"("object in"=w770, "Message"="Zstack", "error in (no error)"=w766) -> ("object out"=w769:refnum<class "Application.lvclass">, "error out"=w767:errorcluster)  [unwired: 15 in]
      }
      event "Zero Z": Value Change {
        n272 = event-data() -> ()  [unwired: 1 in, 6 out]
        n273 = call-dynamic "EnqueueMain.vi"("object in"=w775, "Message"="PriorZero", "error in (no error)"=w771) -> ("object out"=w774:refnum<class "Application.lvclass">, "error out"=w772:errorcluster)  [unwired: 15 in]
      }
      event "Freq Sweep (Ch1)": Value Change {
        n274 = event-data() -> ()  [unwired: 1 in, 6 out]
        n275 = call-dynamic "EnqueueMain.vi"("object in"=w780, "Message"="AD2Configure", "error in (no error)"=w778) -> ("object out"=w779:refnum<class "Application.lvclass">, "error out"=w777:errorcluster)  [unwired: 15 in]
      }
    }
    n276 = call-dynamic "ErrorHandlerEventLoop.vi"("object in"=w568, "error in (no error)"=w570) -> ("object out"=w567:refnum<class "Application.lvclass">, "error out"=w569:errorcluster)  [unwired: 16 in]
  }
  n277 = Merge Errors(w7, w6) -> (w4:errorcluster)
  n278 = call-dynamic "CleanUp.vi"("object in"=w5, "error in (no error)"=w4) -> ()  [unwired: 16 in, 2 out]
